vi "Ladder chip&bias ring encapsulation v1.vi"() -> ()   [LabVIEW 2016]
uses:
  Classes/Controllers/Camera/Copy of Controller Folder/Controller.lvclass
  <vilib>/Utility/file.llb/Read Delimited Spreadsheet (DBL).vi
  Classes/Controllers/Motion/Copy of Motion Folder/Motion.lvclass
  Classes/Controllers/Dispenser/Copy of Ultimus V2 Folder/Ultimus V2.lvclass
  Classes/Controllers/I-O/Copy of NI-DAQ Folder/NI-DAQ.lvclass
  <vilib>/Analysis/NI_AALPro.lvlib
  <vilib>/Analysis/coordinate.llb/2D Cartesian Coordinate Rotation (Scalar).vi
  <vilib>/Utility/file.llb/Write Delimited Spreadsheet (DBL).vi
panel:
  out "Needle parking position 2":dbl[](array[numeric])
  out "x+y 2":dbl[](array[numeric])
  out "corner index 2":i32
  in  "Deposit Glue for chip":bool
  out "Measured HDI size":dbl[](array[numeric])
  out "Measured HDI top left mark":dbl[](array[numeric])
  out "Sample on HDI":dbl[][](array[numeric]) format="%#_8g"
  in  "Default HDI size":dbl[](array[numeric])=[24.2991, 231.315, -0.0249987, -3.34415e-05]
  in  "Default HDI alignment \nmark position":dbl[](array[numeric])=[448.231, 973.808, 78.9737, -3.34415e-05]
  in  "Needle gap for real":dbl=1.3
  out "corner index":i32
  out "Array":dbl[](array[numeric])
  out "x+y":dbl[](array[numeric])
  out "CMC positions":dbl[][][](array[numeric])
  in  "deposit module":i32=2
  out "Stave mark":dbl[][](array[numeric])
  in  "Default Stave dimension":dbl[](array[numeric])=[34.0, 472.0, -0.335295, -0.000320234]
  in  "Default Stave upper left mark":dbl[](array[numeric])=[584.376, 675.576, 70.9882, 0.000840064]
  out "Needle parking position":dbl[](array[numeric])
  in  "Uppler / Lower Stave":bool=TRUE
  out "Gantry current position":dbl[](array[numeric])
  in  "READ Position":bool
  in  "Needle Alignment":bool
  in  "Parking position":dbl[](array[numeric])=[625.0, 625.0, 0.0, 0.01]
  in  "GOTO":bool
  out "# of tasks excuted":i32
  in  "Inititalize":bool
  in  "Deposit Glue for bias ring":bool
  in  "Stop":bool
  in  "Measure HDI":bool
  # "Upper\nmodule"
  # "Lower\nmodule"
  # "Chip & Bias ring encapsulation"
  # "Module infomation"
  # "before \"HDI cornrer\" click \"Initialize\""
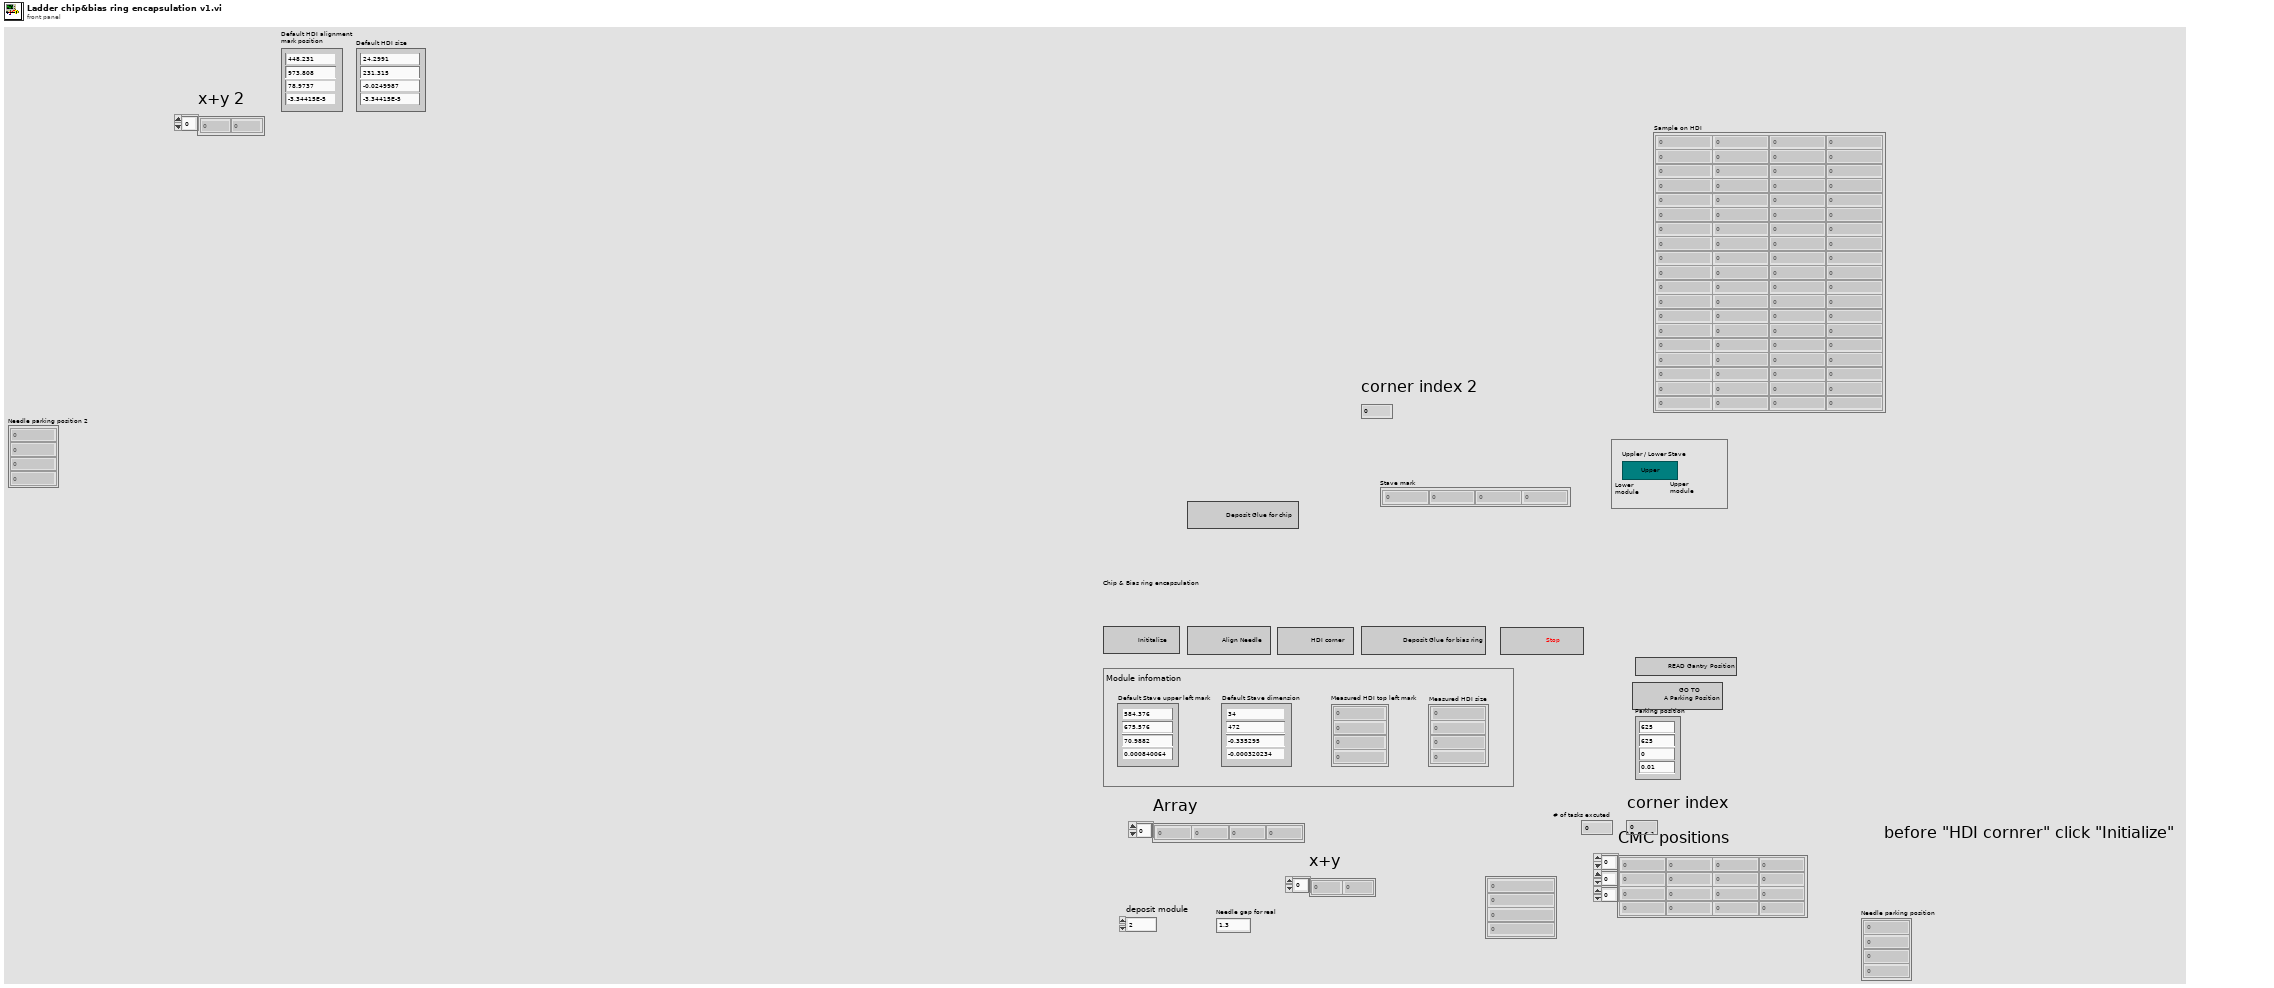
[diagram p1: front panel]
types:
  T1 = typedef "Controller.lvclass/Controllers.ctl" = cluster{"Copy of Motion.lvclass":refnum<class "Motion.lvclass">, "Copy of I-O.lvclass":refnum<class "I-O.lvclass">, "Copy of Dispenser.lvclass":refnum<class "Dispenser.lvclass">}
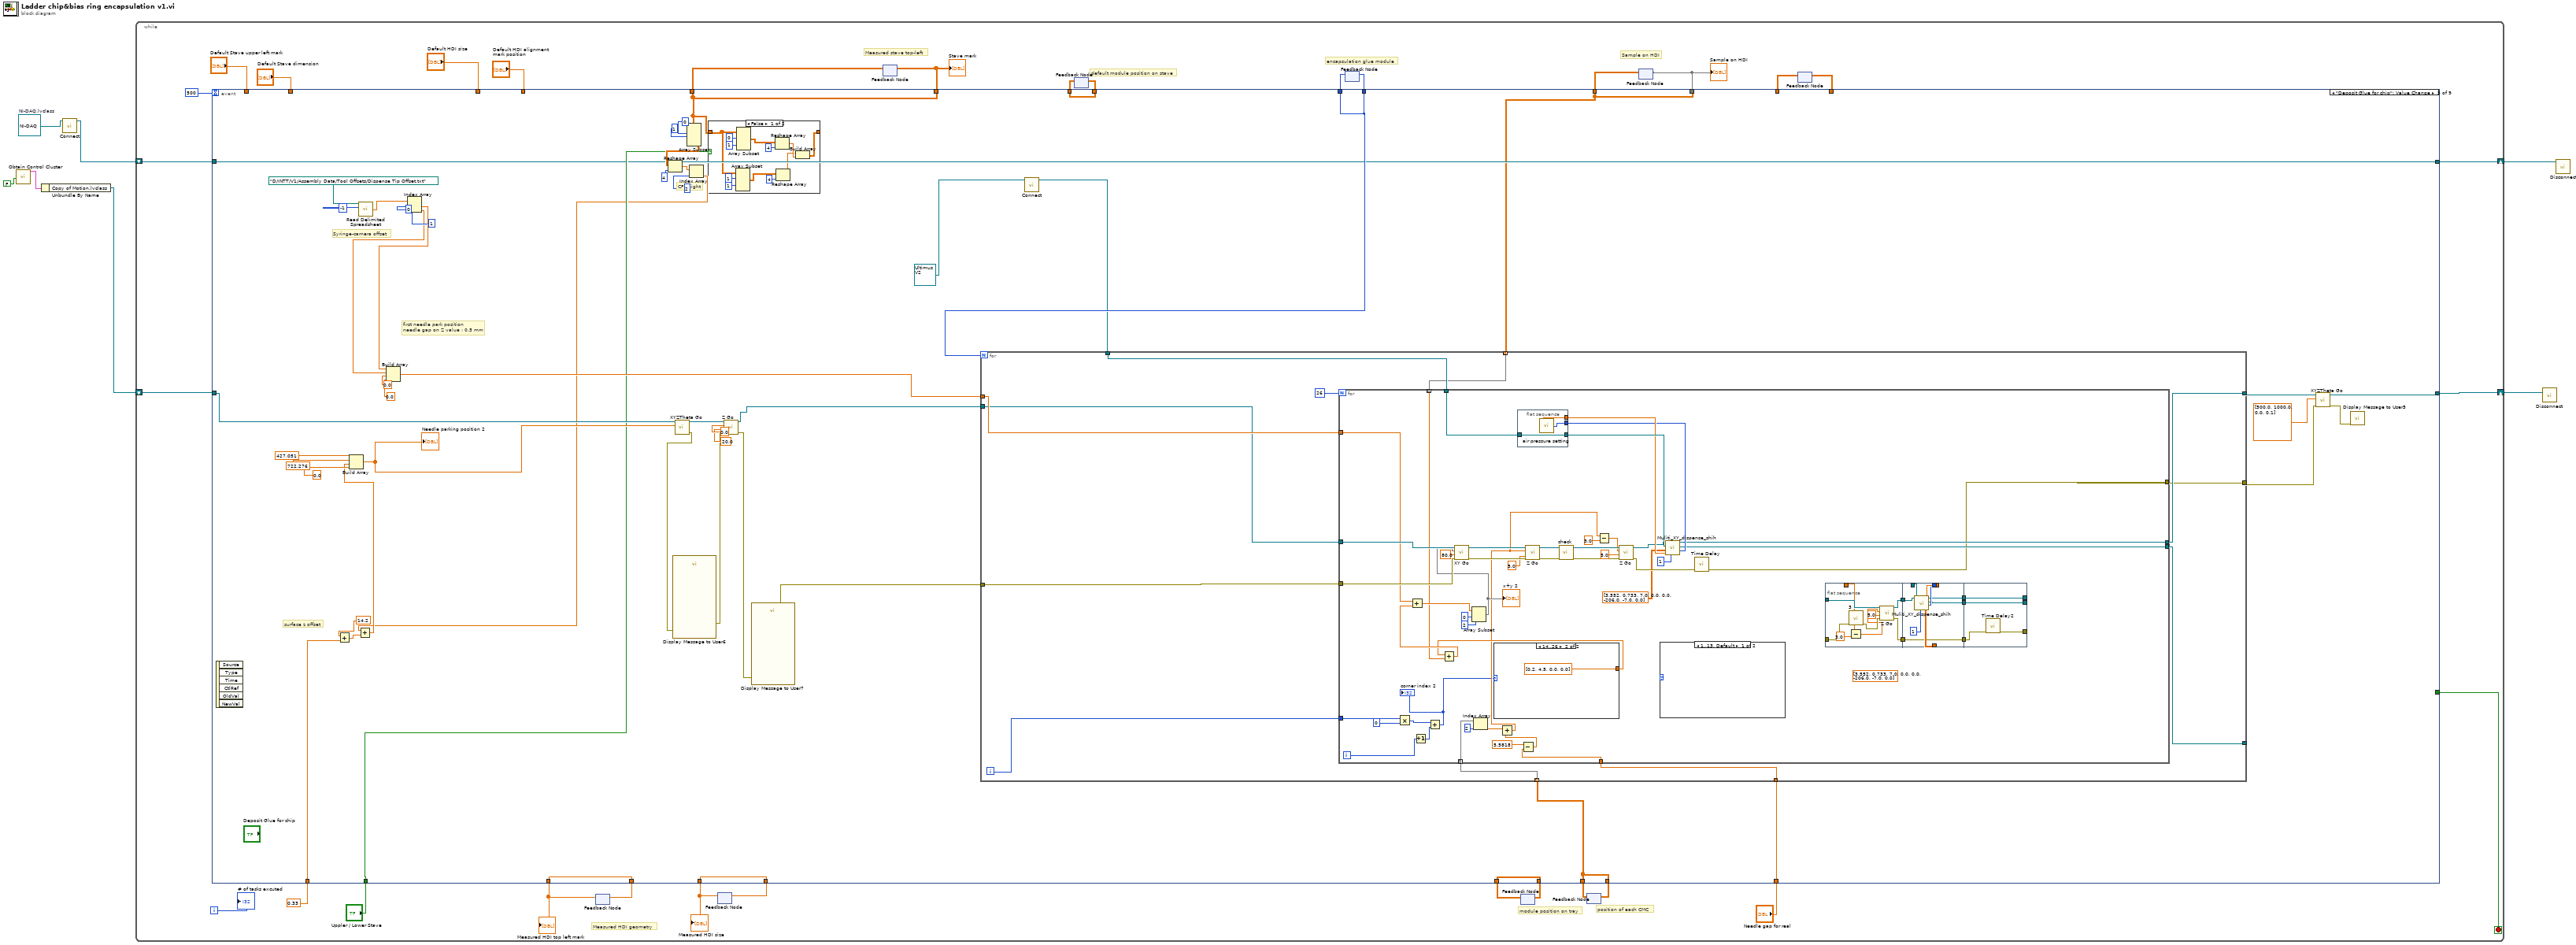
[diagram p0: block diagram]
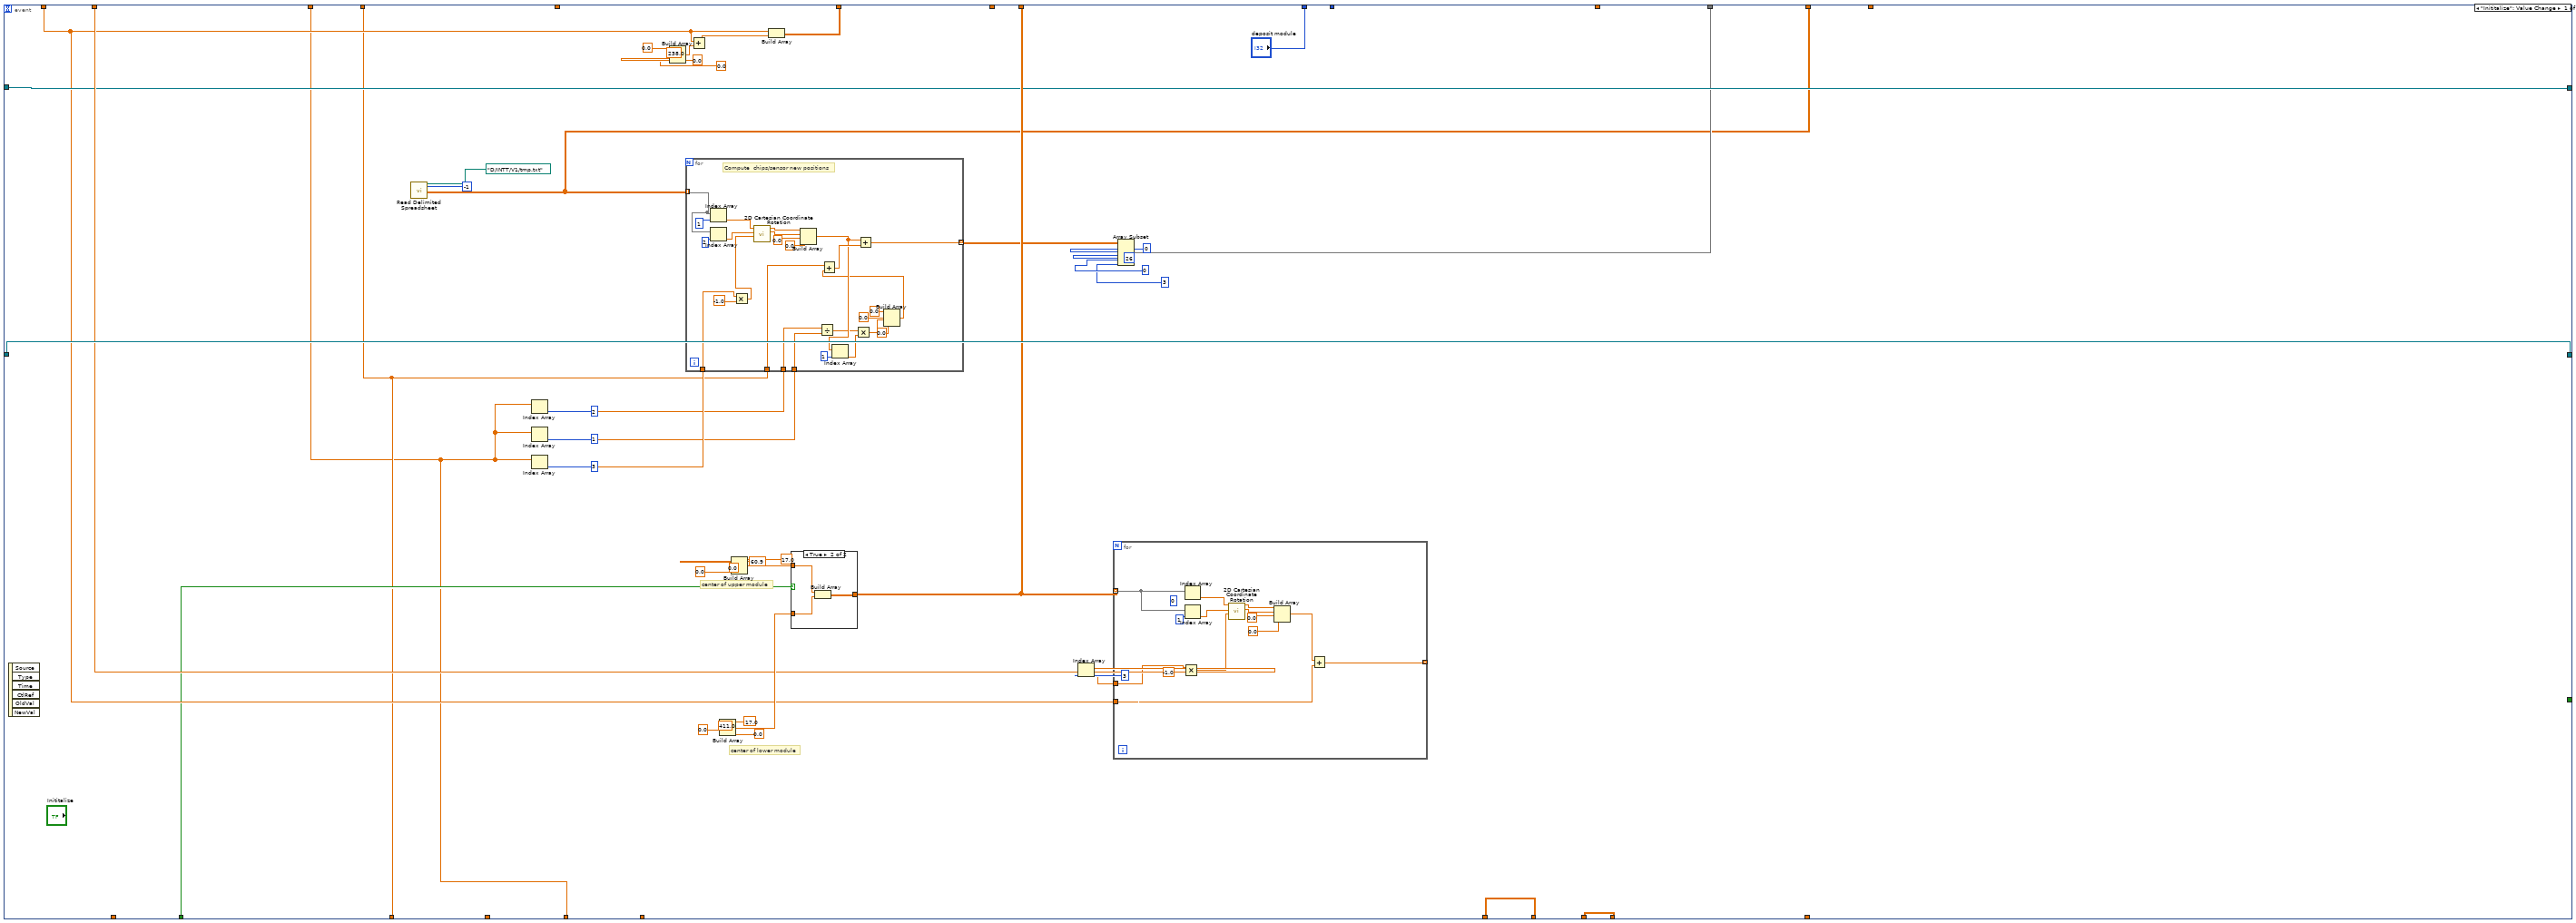
[diagram p2: hidden frame]
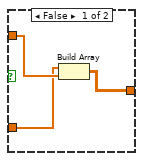
[diagram p3: hidden frame]
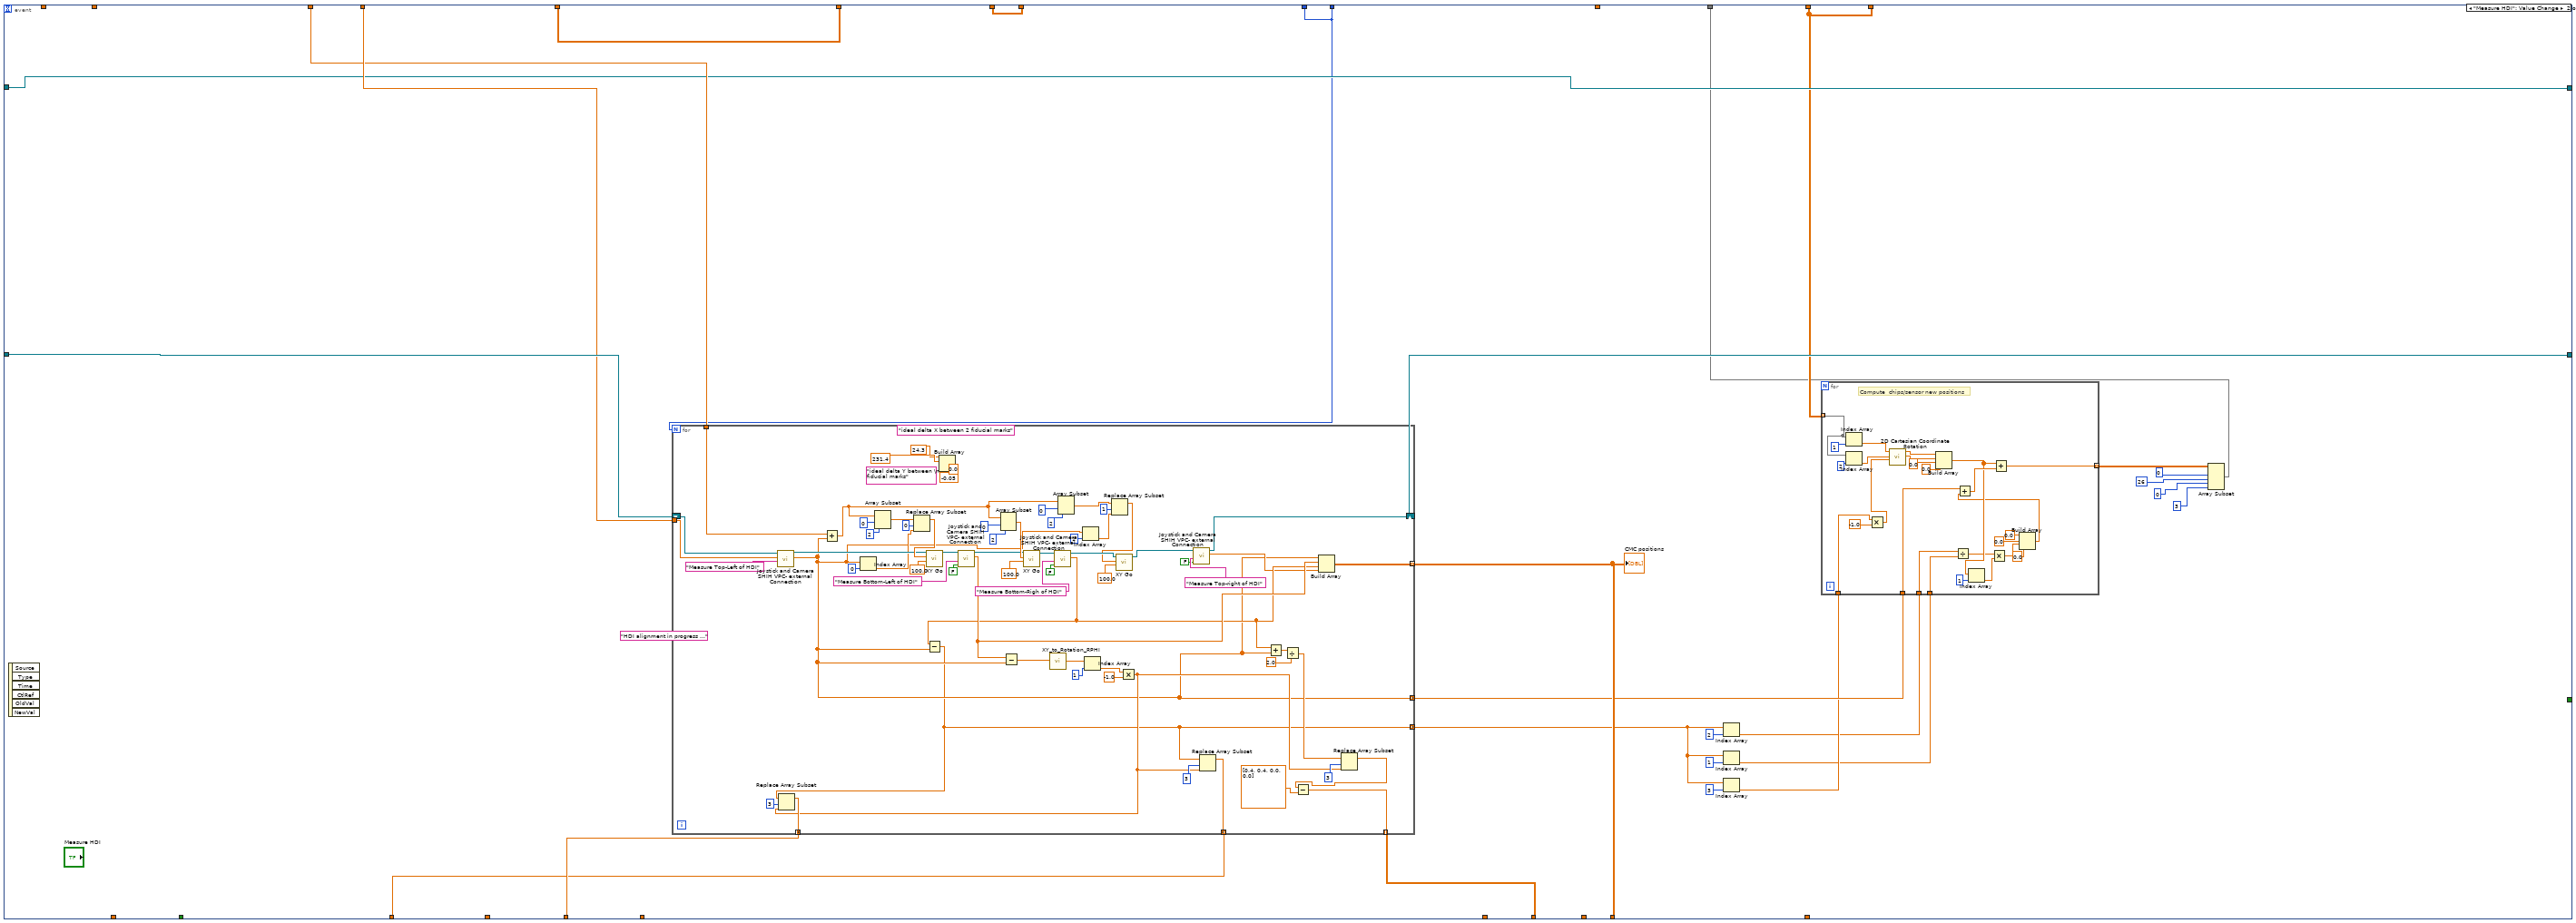
[diagram p4: hidden frame]
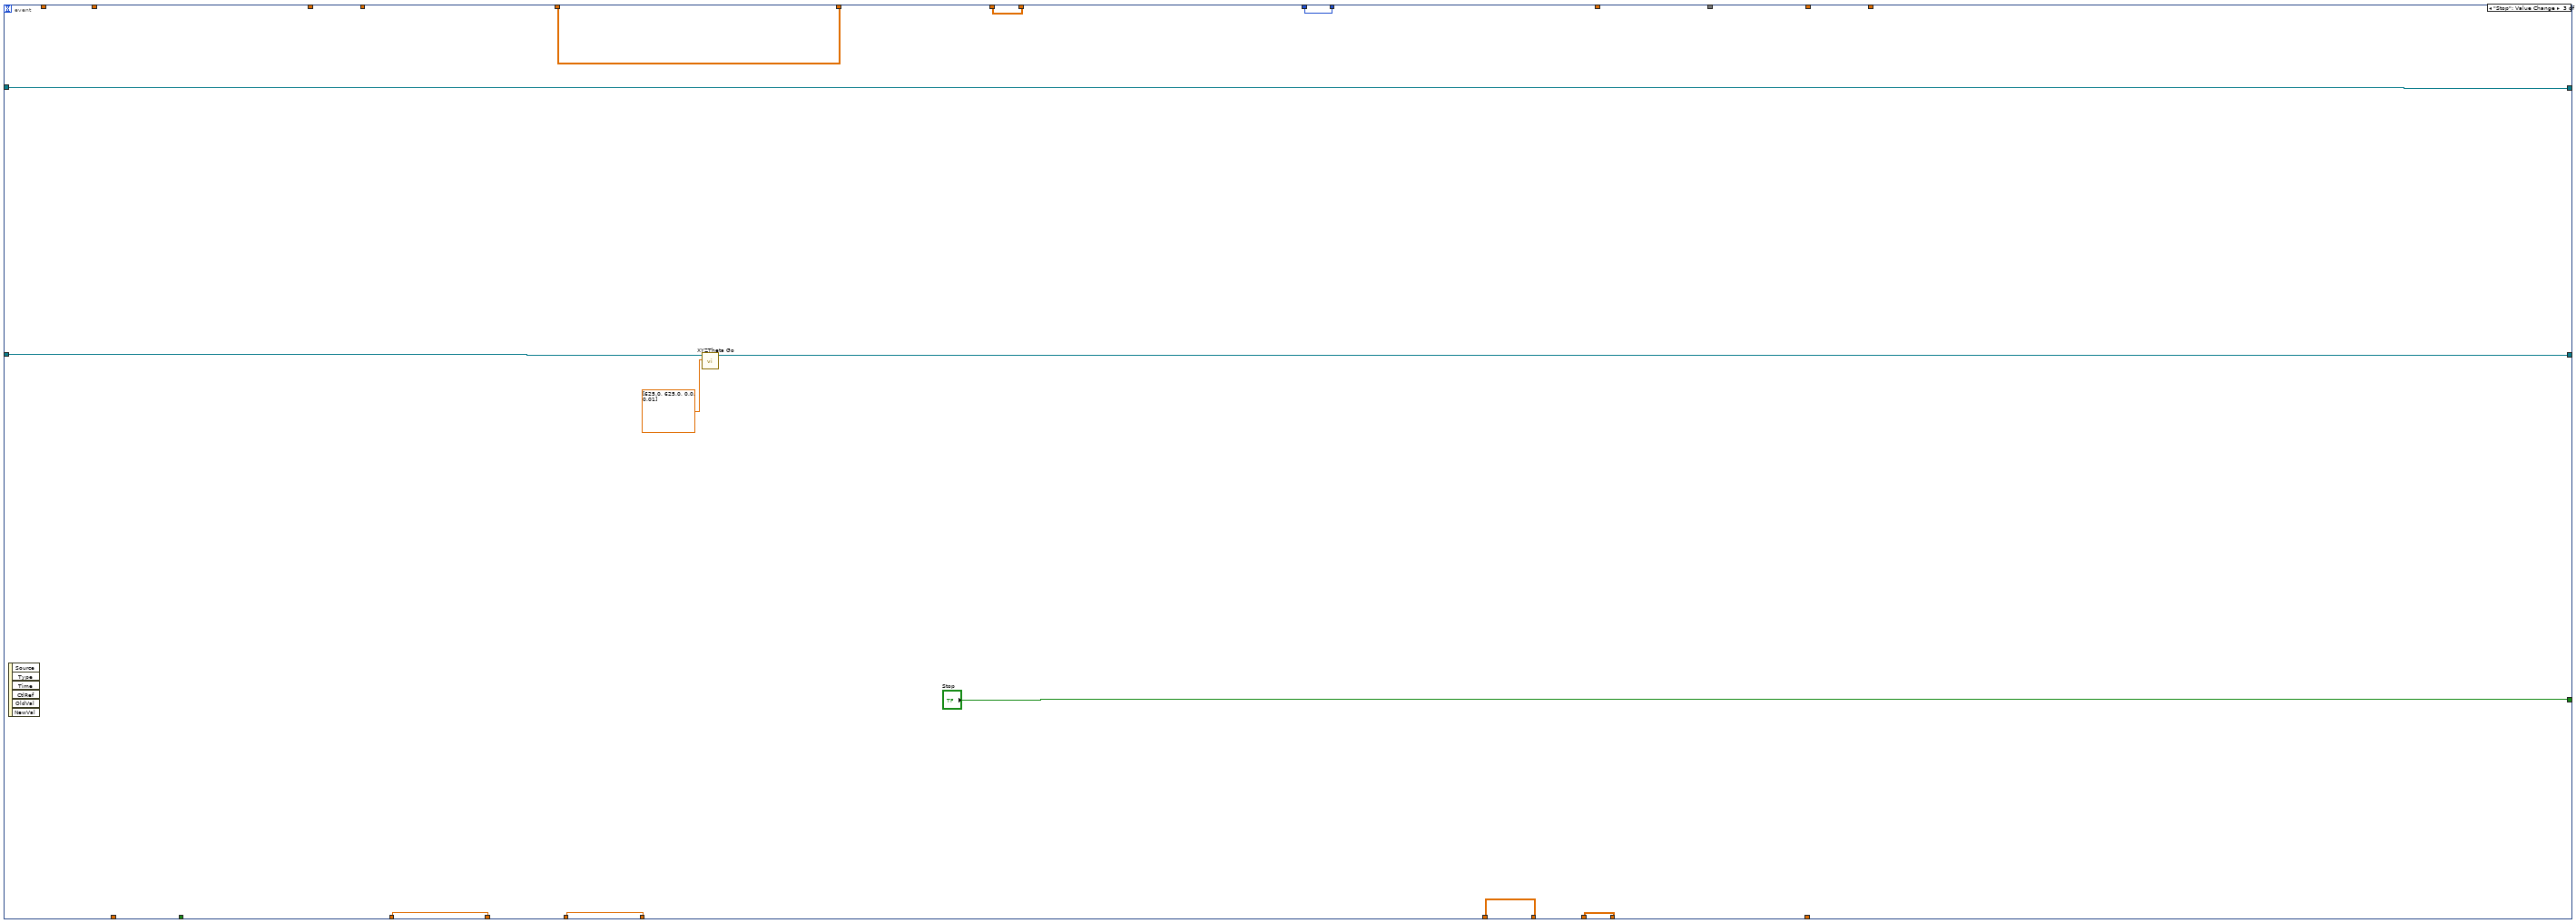
[diagram p5: hidden frame]
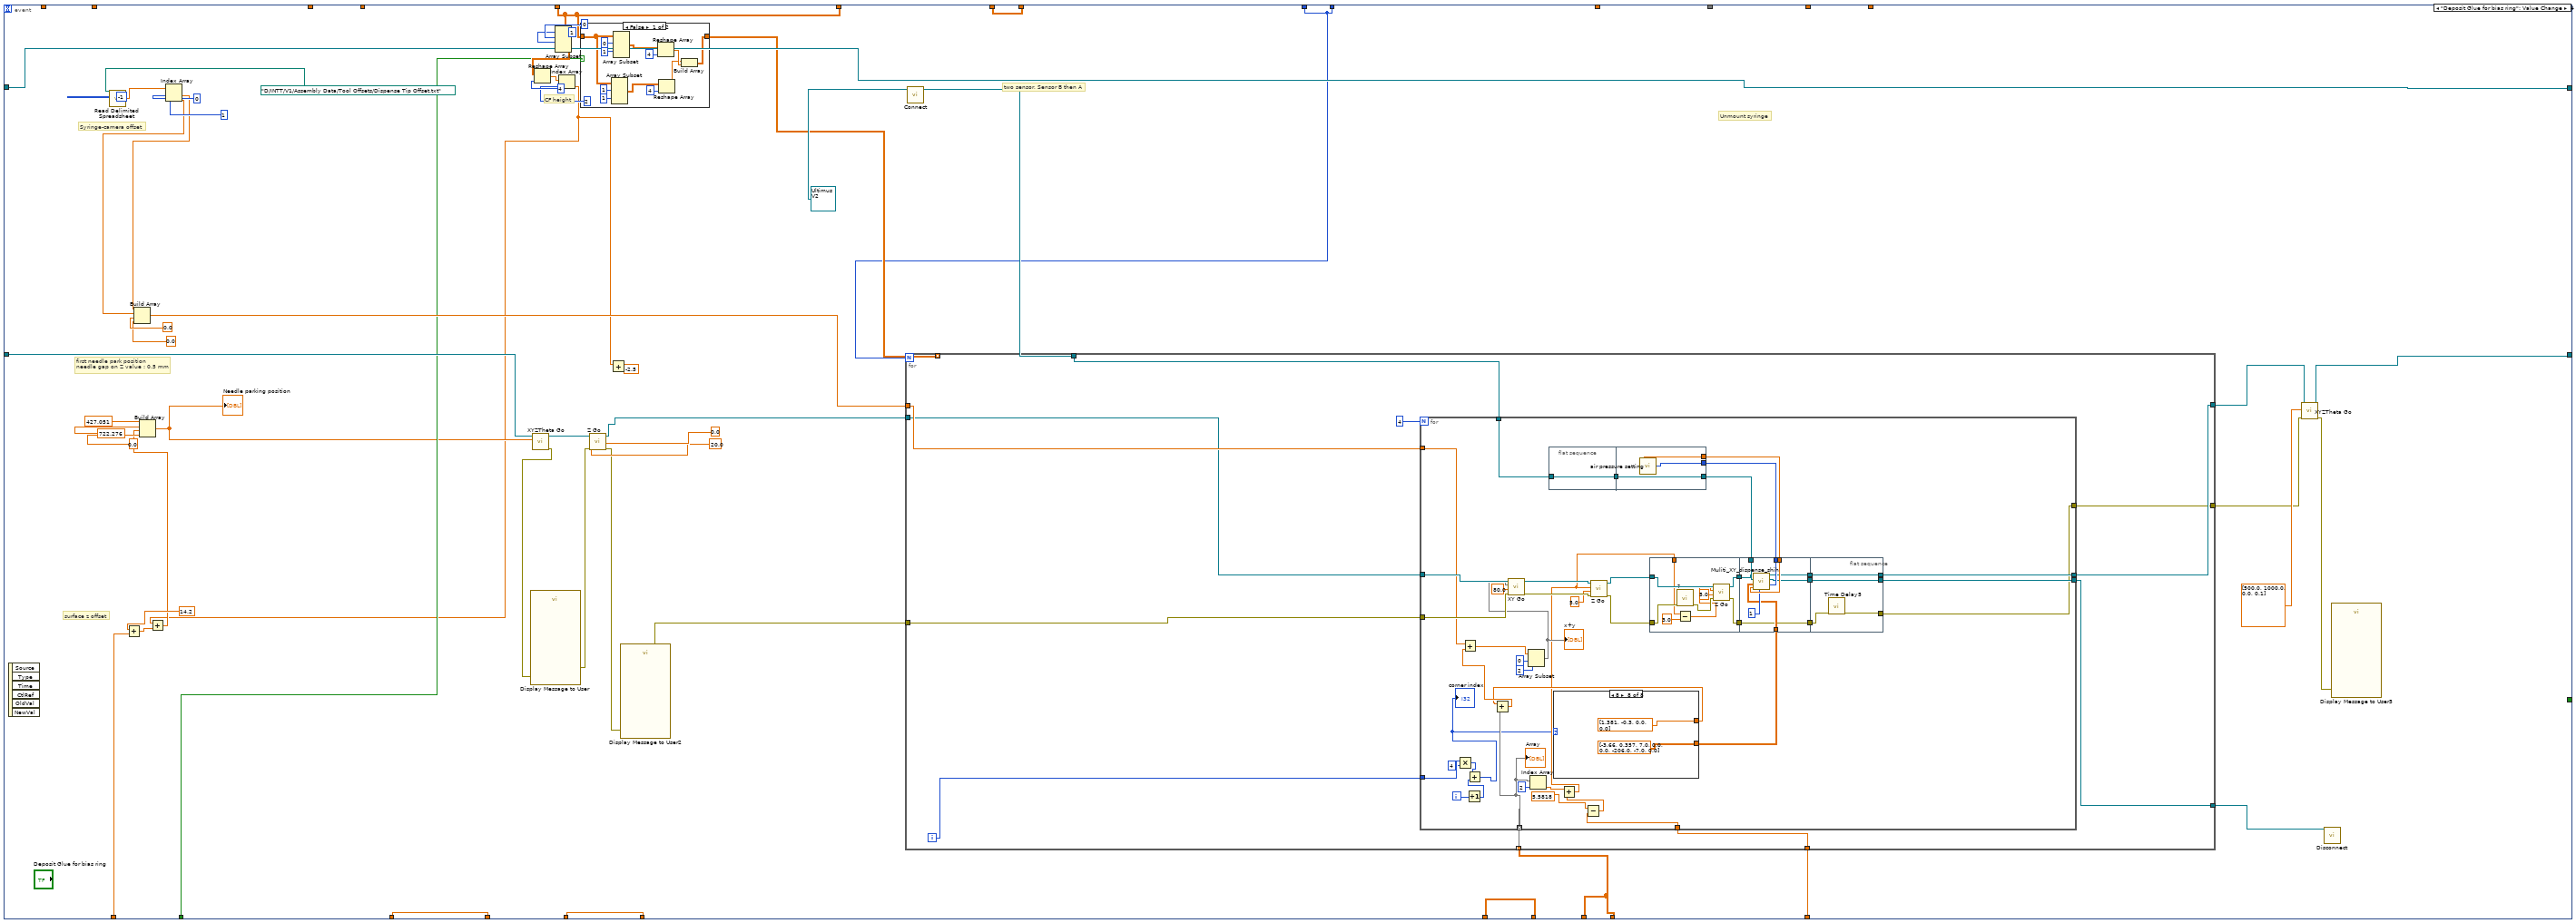
[diagram p6: hidden frame]
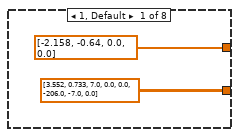
[diagram p8: hidden frame]
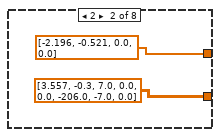
[diagram p9: hidden frame]
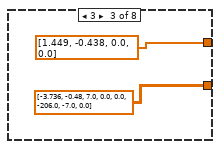
[diagram p10: hidden frame]
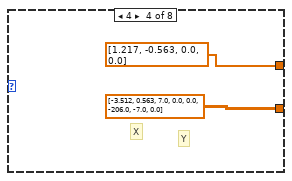
[diagram p11: hidden frame]
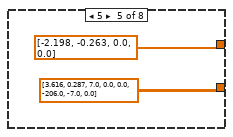
[diagram p12: hidden frame]
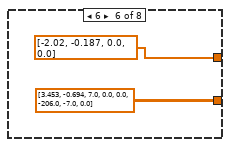
[diagram p13: hidden frame]
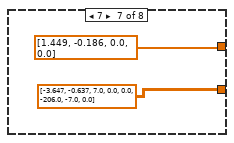
[diagram p14: hidden frame]
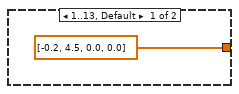
[diagram p17: hidden frame]
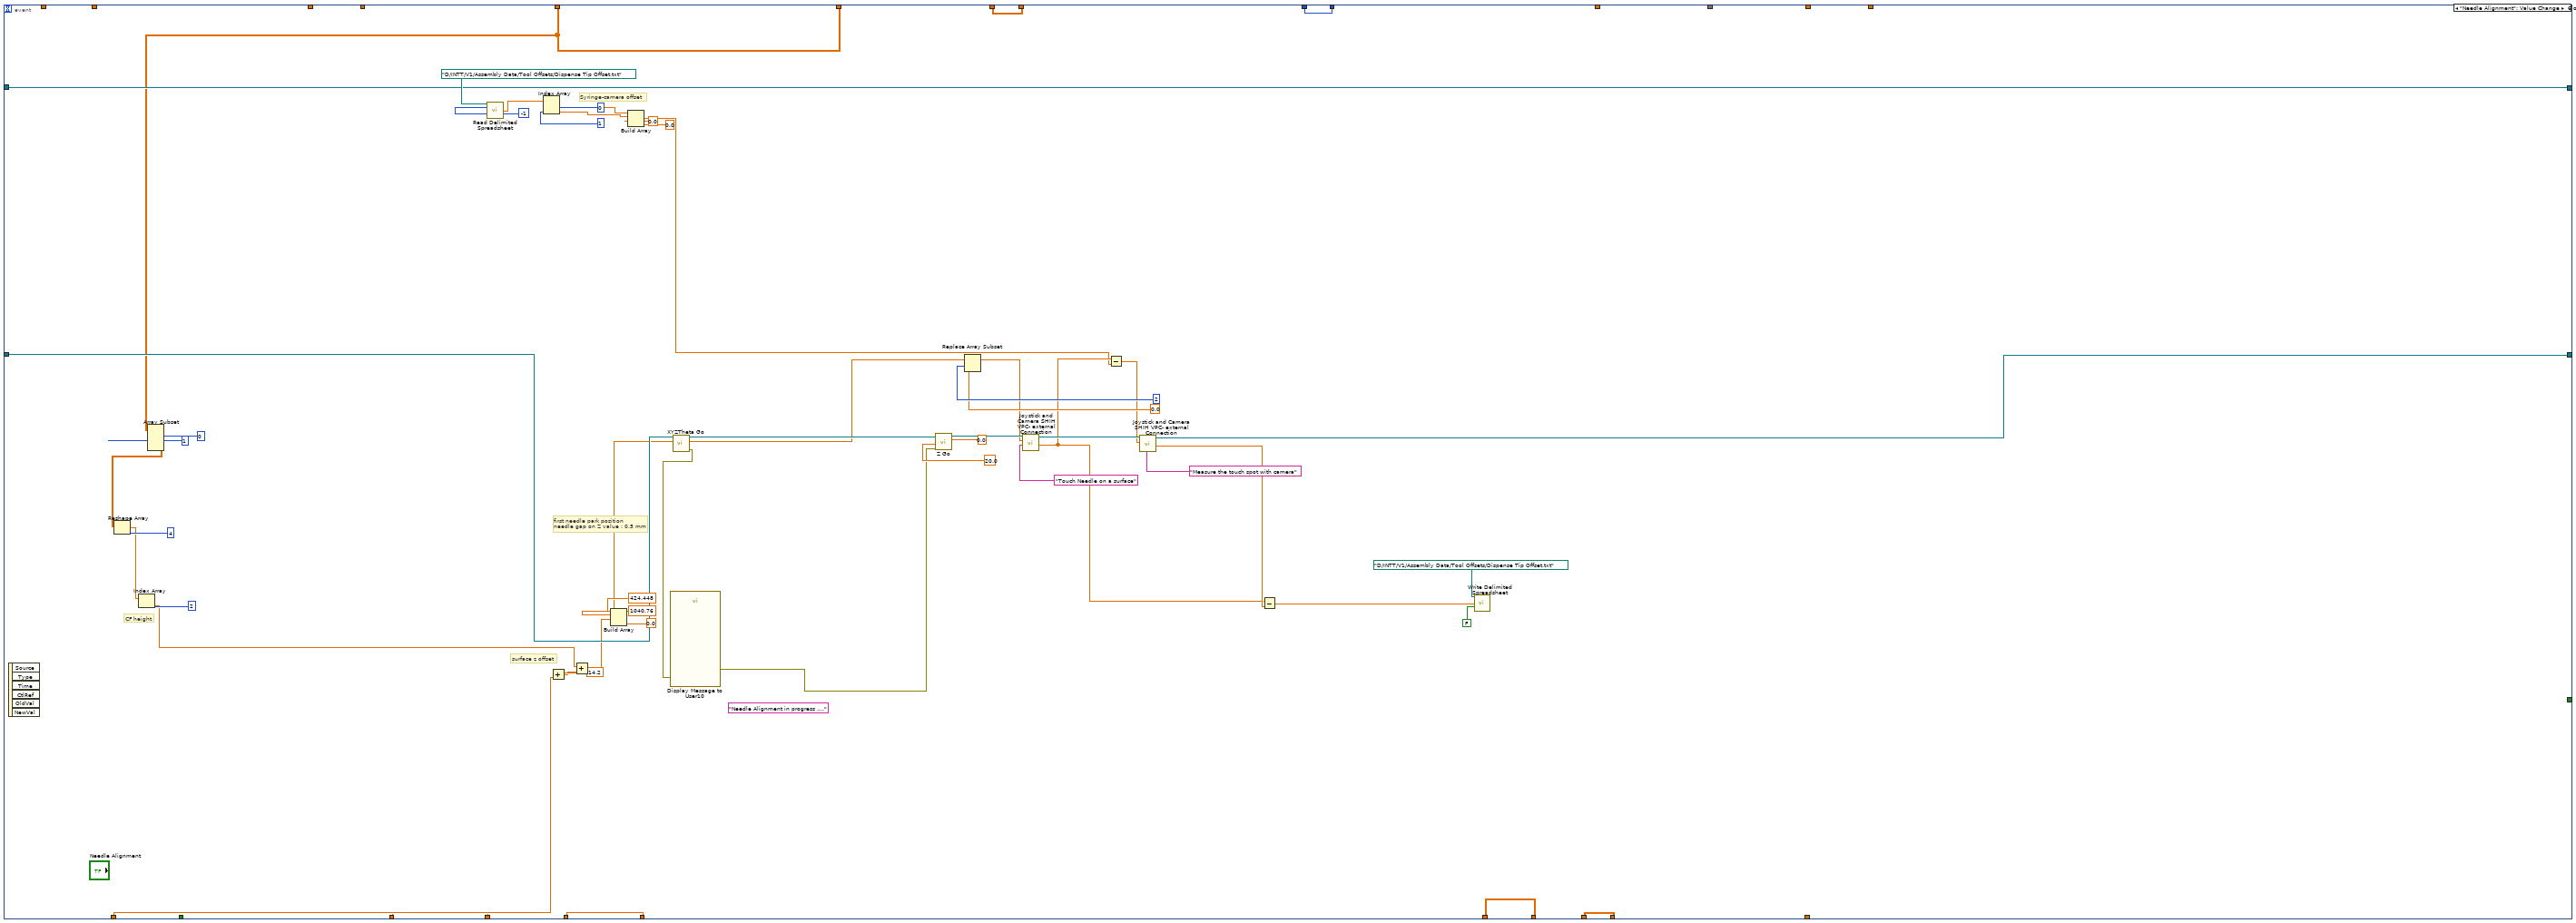
[diagram p18: hidden frame]
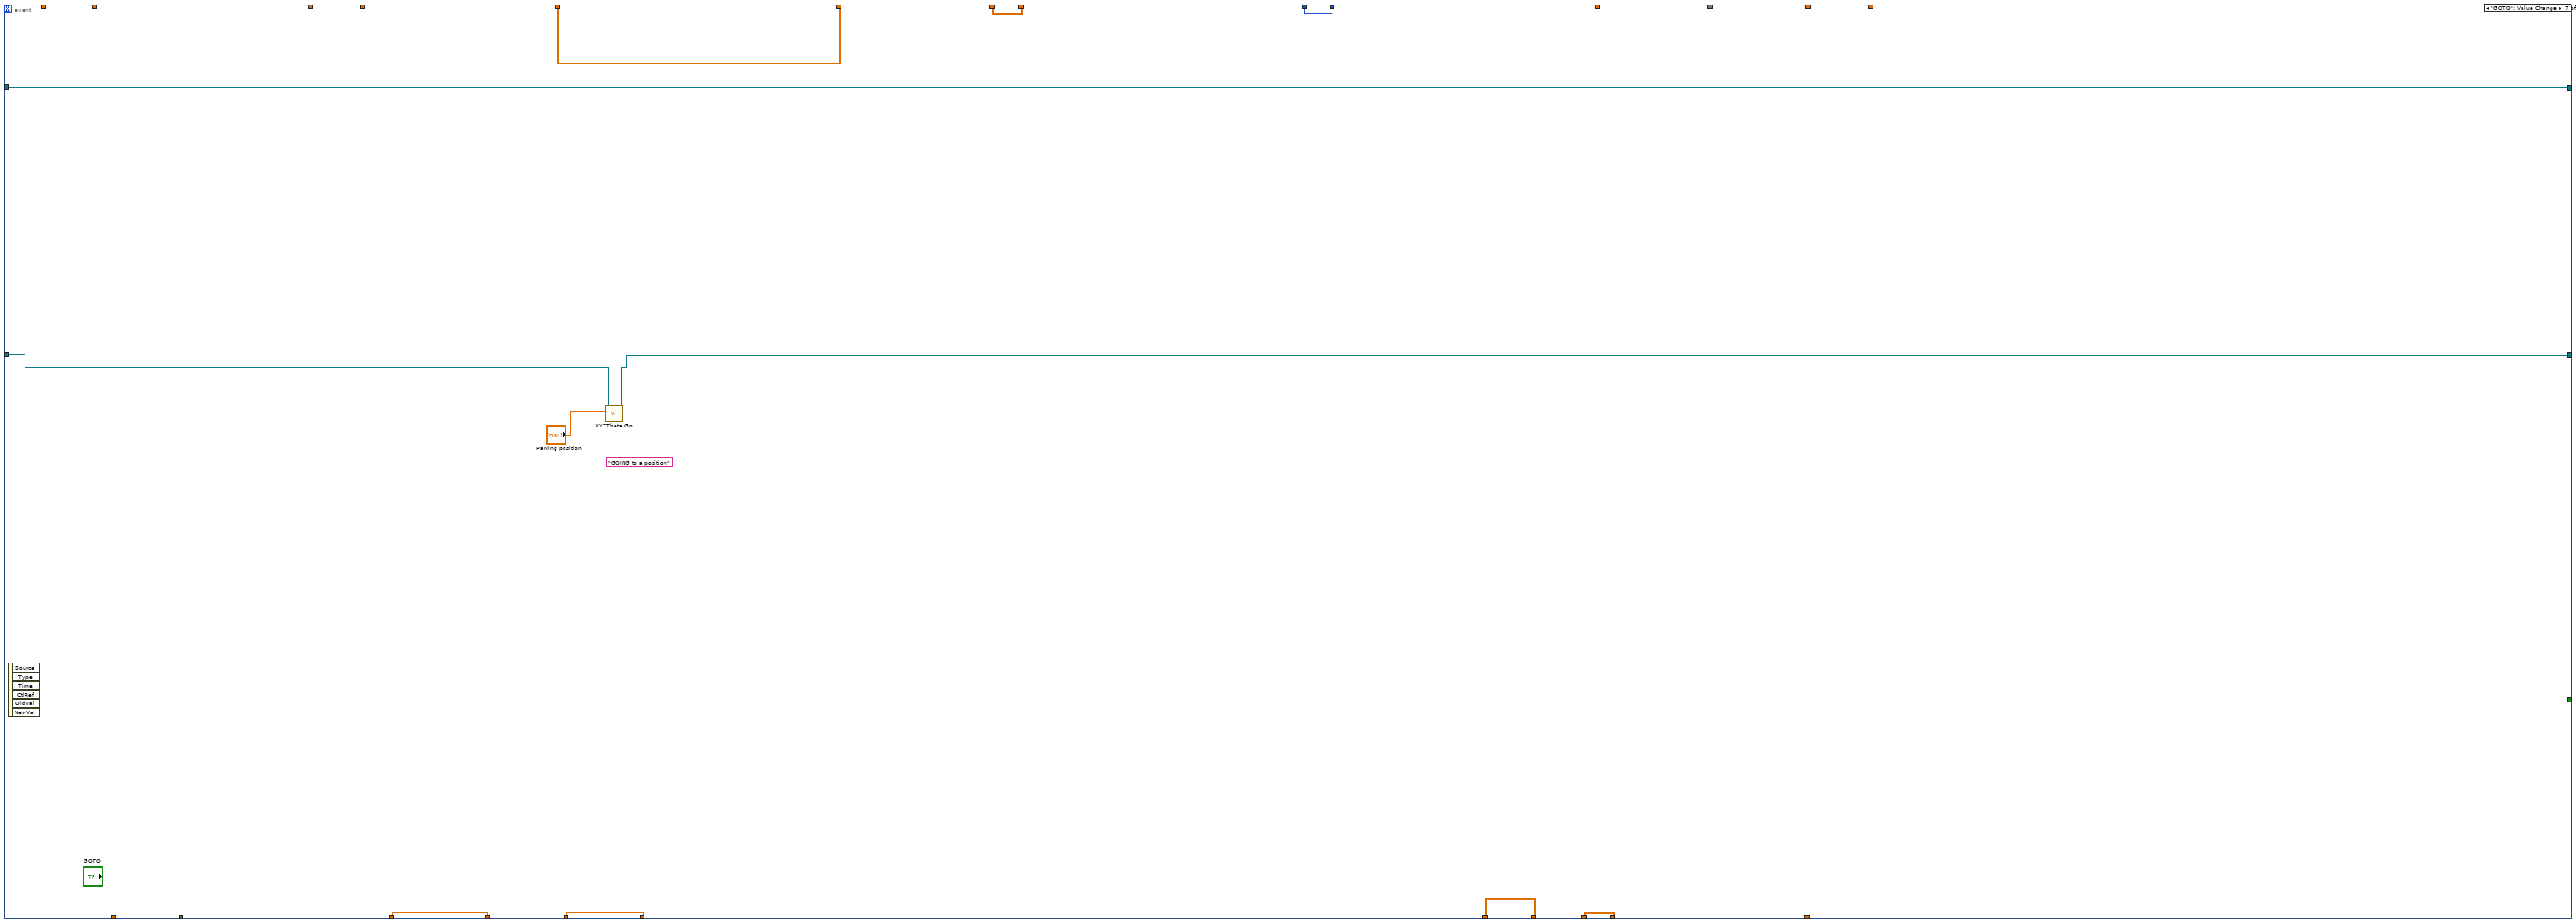
[diagram p19: hidden frame]
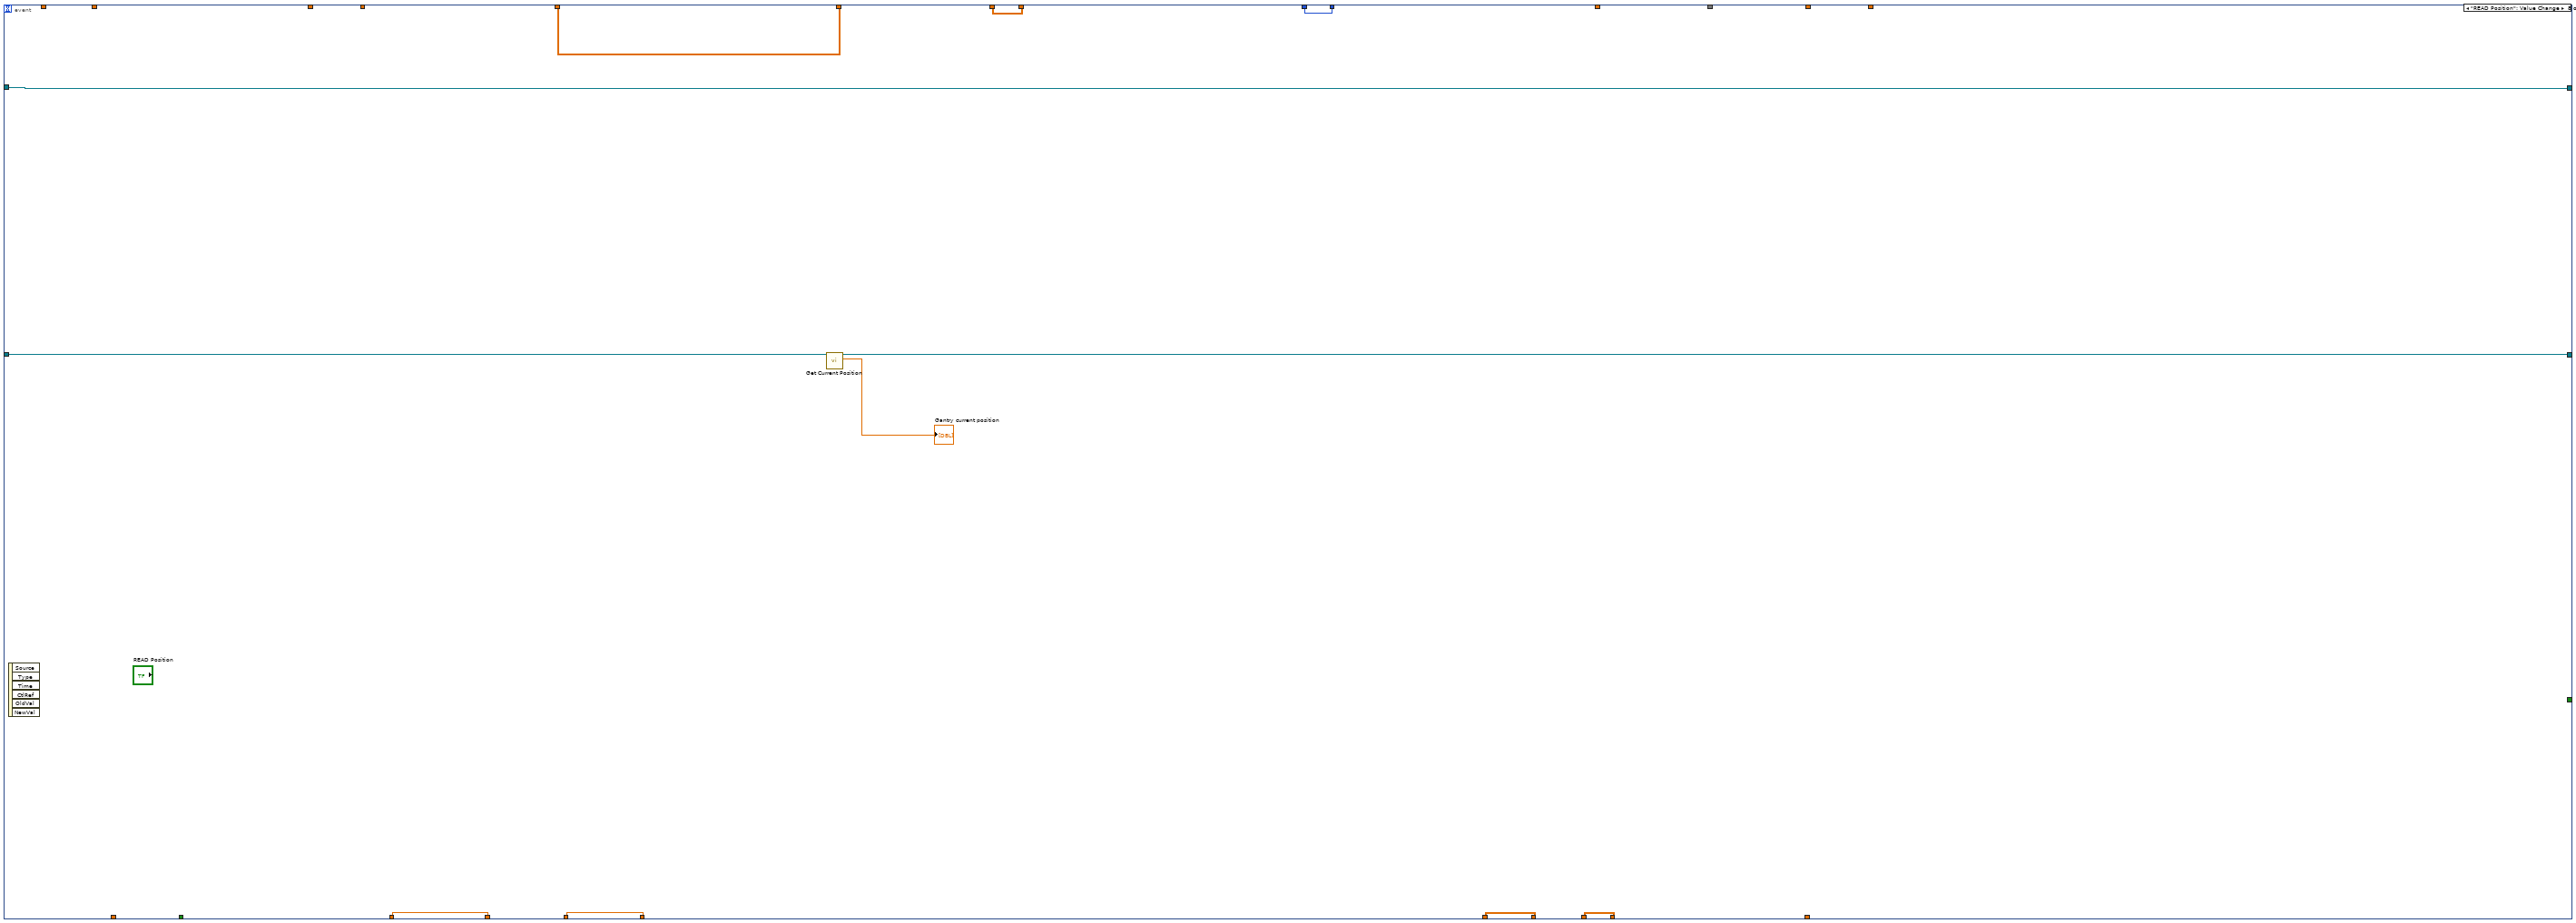
[diagram p20: hidden frame]
diagram:
  w3 = refnum<class "NI-DAQ.lvclass"> refnum  # NI-DAQ.lvclass
  n1 = call "Obtain Control Cluster.vi"("I/O"=FALSE) -> ("Control Out"=w7:T1)  [unwired: 10 in]
  n2 = Unbundle By Name(w7) -> ("Copy of Motion.lvclass"=w5:refnum<class "Motion.lvclass">)
  n3 = call-dynamic "Connect.vi"("NI-DAQ in"=w3) -> ("NI-DAQ out"=w2:refnum<class "NI-DAQ.lvclass">)  [unwired: 9 in, 1 out]
  n4 = while {
    shift-right: [w34] -> w4
    shift-left: w5 -> [w39]
    shift-right: [w24] -> w1
    shift-left: w2 -> [w26]
    i -> [w33]
    stop <- w38 stop-if-true
    # "Sample on HDI"
    # "position of each CMC"
    # "encapsulation glue module"
    # "default module position on stave"
    # "Measured HDI geometry"
    # "module position on tray"
    # "Measured stave top-left"
    n5 = feedback #1() -> (w25:dbl[])  [unwired: 1 in]
    n6 = feedback #2() -> (w36:dbl[])  [unwired: 1 in]
    n7 = feedback #3() -> (w37:dbl[][])  [unwired: 1 in]
    n8 = feedback #4() -> (w31:dbl[][])  [unwired: 1 in]
    n9 = feedback #5() -> (w19:i32)  [unwired: 1 in]
    n10 = feedback #6() -> (w21:dbl[][])  [unwired: 1 in]
    n11 = feedback #7() -> (w17:dbl[][][])  [unwired: 1 in]
    n12 = feedback #8() -> (w12:dbl[][])  [unwired: 1 in]
    n13 = feedback #9() -> (w8:dbl[][])  [unwired: 1 in]
    n14 = event shown="[4] \"Deposit Glue for chip\": Value Change" {
      selector: _ -> [_ _ _ _ _ _ _ _ _]
      dyn-events: _ -> [_ _ _ _ _ _ _ _ _]
      timeout: 500 -> [_ _ _ _ _ _ _ _ _]
      tunnel: w39 -> [w84 w157 w260 w297 w448 w613 w637 w651 w659]
      tunnel: [_ _ "Stop" _ _ _ _ _ _] -> w38
      tunnel: [w60 w152 w256 w269 w434 w581 w640 w648 w658] -> w27
      tunnel: w37 -> [_ w152 w256 w269 w434 w581 w640 w648 w658]
      tunnel: w36 -> [_ _ w249 w261 w425 w576 w630 w641 w653]
      tunnel: [w70 w151 w255 w288 w427 w614 w638 w647 w656] -> w35
      tunnel: w21 -> [w70 _ w255 w288 w427 w614 w638 w647 w656]
      tunnel: [w84 w156 w258 w289 w462 w605 w635 w650 w659] -> w34
      tunnel: "Default HDI alignment \nmark position" -> [w42 w155 _ _ _ _ _ _ _]
      tunnel: "Default HDI size" -> [w41 w154 _ _ _ _ _ _ _]
      tunnel: [w73 w153 w257 w287 w424 w615 w639 w649 w657] -> w32
      tunnel: w31 -> [_ w153 w257 w287 w424 w615 w639 w649 w657]
      tunnel: "Uppler / Lower Stave" -> [w57 _ _ w277 w433 _ _ _ _]
      tunnel: "Default Stave upper left mark" -> [w61 _ _ _ _ _ _ _ _]
      tunnel: "Default Stave dimension" -> [w69 _ _ _ _ _ _ _ _]
      tunnel: w26 -> [w68 w150 w253 w283 w430 w596 w634 w645 w661]
      tunnel: [w68 w150 w253 w283 w430 w596 w634 w645 w660] -> w24
      tunnel: w25 -> [_ _ w250 w262 w426 w577 w631 w642 w652]
      tunnel: 0.33 ("Needle Height Compenstation\n(glue gap)") -> [_ _ _ w278 w431 w589 _ _ _]
      tunnel: ["deposit module" w149 w252 w267 w459 w579 w633 w644 w655] -> w20
      tunnel: w19 -> [_ w149 w252 w267 w459 w579 w633 w644 w655]
      tunnel: [w58 w148 w251 w263 w428 w578 w632 w643 w654] -> w18
      tunnel: w17 -> [w58 _ w251 w263 w428 w578 w632 w643 w654]
      tunnel: "Needle gap for real" -> [_ _ _ w264 w429 _ _ _ _]
      tunnel: [w43 w131 _ _ w423 _ _ _ _] -> w13
      tunnel: w12 -> [_ _ _ _ w423 _ _ _ _]
      tunnel: [w42 w146 w250 w262 w426 w577 w631 w642 w652] -> w11
      tunnel: [w41 w147 w249 w261 w425 w576 w630 w641 w653] -> w10
      tunnel: [w40 w145 _ _ _ _ _ _ _] -> w9
      tunnel: w8 -> [_ w145 _ _ _ _ _ _ _]
      event "Inititalize": Value Change {
        # "center of lower module"
        # "center of upper module"
        n15 = event-data() -> ()  [unwired: 1 in, 6 out]
        n16 = call-poly <vilib>:"Read Delimited Spreadsheet.vi"("file path (dialog if empty)"=path "D:/INTT/V1/tmp.txt", "number of rows (all:-1)"=-1) -> ("all rows"=w40:dbl[][])  [unwired: 8 in, 5 out]
        n17 = Index Array(array=w41, index=2) -> (element=w49:dbl)
        n18 = Index Array(array=w41, index=1) -> (element=w50:dbl)
        n19 = Index Array(array=w41, index=3) -> (element=w51:dbl)
        n20 = Build Array(0.0 ("element"), 238.0 ("element"), 0.0 ("element"), 0.0 ("element")) -> (w63:dbl[])
        n21 = for {
          tunnel: w40 -> [w103] mode=indexing
          tunnel: w51 -> [w88]
          tunnel: w42 -> [w96]
          tunnel: [w102] -> w44 mode=indexing
          tunnel: w49 -> [w101]
          tunnel: w50 -> [w94]
          # "Compute  chips/sensor new positions"
          n22 = Index Array(array=w103, index=1) -> (element=w107:dbl)
          n23 = Index Array(array=w103, index=2) -> (element=w106:dbl)
          n24 = Multiply(x=w88, y=-1.0) -> (x*y=w89:dbl)
          n25 = call-poly <vilib>:"2D Cartesian Coordinate Rotation.vi"("theta"=w89, "y"=w106, "x"=w107) -> ("y out"=w109:dbl, "x out"=w108:dbl)  [unwired: 6 in, 1 out]
          n26 = Build Array(w108, w109, 0.0 ("element"), 0.0 ("element")) -> (w91:dbl[])
          n27 = Divide(x=w101, y=w94) -> (x/y=w85:dbl)
          n28 = Index Array(array=w91, index=1) -> (element=w92:dbl)
          n29 = Multiply(x=w85, y=w92) -> (x*y=w97:dbl)
          n30 = Build Array(0.0 ("element"), 0.0 ("element"), w97, 0.0 ("element")) -> (w86:dbl[])
          n31 = Add(x=w96, y=w86) -> (x+y=w95:dbl[])
          n32 = Add(x=w91, y=w95) -> (x+y=w102:dbl[])
        }
        n33 = Add(x=w61, y=w63) -> (x+y=w62:dbl[])
        n34 = Build Array(17.0 ("element"), 411.0 ("element"), 0.0 ("element"), 0.0 ("element")) -> (w74:dbl[])
        n35 = Build Array(17.0 ("element"), 60.9 ("element"), 0.0 ("element"), 0.0 ("element")) -> (w75:dbl[])
        n36 = Build Array(w61, w62) -> (w60:dbl[][])
        n37 = case shown="True" w57 {
          tunnel: w75 -> [w113 w116]
          tunnel: w74 -> [w112 w115]
          tunnel: [w111 w114] -> w73
          frame False {
            n38 = Build Array(w112, w113) -> (w111:dbl[][])
          }
          frame True {
            n39 = Build Array(w116, w115) -> (w114:dbl[][])
          }
        }
        n40 = Index Array(array=w69, index=3) -> (element=w71:dbl)
        n41 = for {
          tunnel: w73 -> [w124] mode=indexing
          tunnel: w71 -> [w118]
          tunnel: w61 -> [w123]
          tunnel: [w121] -> _ mode=indexing
          (unwired) 0 ("index")
          n42 = Multiply(x=w118, y=-1.0) -> (x*y=w119:dbl)
          n43 = Index Array(array=w124) -> (element=w127:dbl)  [unwired: 1 in]
          n44 = Index Array(array=w124, index=1) -> (element=w126:dbl)
          n45 = call-poly <vilib>:"2D Cartesian Coordinate Rotation.vi"("theta"=w119, "y"=w126, "x"=w127) -> ("y out"=w129:dbl, "x out"=w128:dbl)  [unwired: 6 in, 1 out]
          n46 = Build Array(w128, w129, 0.0 ("element"), 0.0 ("element")) -> (w122:dbl[])
          n47 = Add(x=w122, y=w123) -> (x+y=w121:dbl[])
        }
        n48 = Array Subset(array=w44, index (row)=0 ("index"), length (row)=26 ("length"), index (col)=0, length (col)=3 ("length")) -> (w43:dbl[][])
      }
      event "Measure HDI": Value Change {
        (unwired) "HDI alignment in progress ..." ("String")
        n49 = event-data() -> ()  [unwired: 1 in, 6 out]
        n50 = for {
          N: w149 -> [_]
          tunnel: w154 -> [w213]
          shift-right: [w203] -> w156
          shift-left: w157 -> [w211]
          tunnel: w155 -> [w212]
          tunnel: [w245] -> w146 mode=concatenating
          tunnel: [w244] -> w147 mode=concatenating
          tunnel: [w204] -> w151 mode=indexing
          tunnel: [w186] -> w148 mode=indexing
          tunnel: [w185] -> w144 mode=concatenating
          tunnel: [w184] -> w140 mode=concatenating
          (unwired) "ideal delta Y between \n2 fiducial marks"
          (unwired) "ideal delta X between 2 fiducial marks"
          n51 = call "Joystick and Camera SHIH VPC- external Connection.vi"("Motion in"=w211, "XYZTheta"=w212, "Measurement Point"="Measure Top-Left of HDI") -> ("Motion out"=w225:refnum<class "Motion.lvclass">, "Sum"=w185:dbl[])  [unwired: 4 in, 2 out]
          n52 = Add(x=w213, y=w185) -> (x+y=w196:dbl[])
          n53 = Index Array(array=w185, index=0) -> (element=w216:dbl)
          n54 = Array Subset(array=w196, index=0, length=2) -> (w228:dbl[])
          n55 = Replace Array Subset(array=w228, new element=w216, index=0) -> (w226:dbl[])
          n56 = call-dynamic "XY Go.vi"("Speed"=100.0, "XY"=w226, "Motion in"=w225) -> ("Motion out"=w232:refnum<class "Motion.lvclass">)  [unwired: 7 in, 1 out]
          n57 = Build Array(24.3 ("y"), 231.4 ("y"), 0.0 ("element"), -0.05 ("element")) -> ()  [unwired: 1 out]
          n58 = call "Joystick and Camera SHIH VPC- external Connection.vi"("Motion in"=w232, "Measurement Point"="Measure Bottom-Left of HDI", "Inital GO"=FALSE) -> ("Motion out"=w224:refnum<class "Motion.lvclass">, "Sum"=w189:dbl[])  [unwired: 4 in, 2 out]
          n59 = Array Subset(array=w196, index=0, length=2) -> (w238:dbl[])
          n60 = Subtract(x=w189, y=w185) -> (x-y=w223:dbl[])
          n61 = call-dynamic "XY Go.vi"("Speed"=100.0, "XY"=w238, "Motion in"=w224) -> ("Motion out"=w242:refnum<class "Motion.lvclass">)  [unwired: 7 in, 1 out]
          n62 = call "XY_to_Rotation_RPHI.vi"("X-Y"=w223) -> ("r-phi"=w219:dbl[])
          n63 = call "Joystick and Camera SHIH VPC- external Connection.vi"("Motion in"=w242, "Measurement Point"="Measure Bottom-Righ of HDI", "Inital GO"=FALSE) -> ("Motion out"=w201:refnum<class "Motion.lvclass">, "Sum"=w188:dbl[])  [unwired: 4 in, 2 out]
          n64 = Subtract(x=w188, y=w185) -> (x-y=w184:dbl[])
          n65 = Array Subset(array=w196, index=0, length=2) -> (w192:dbl[])
          n66 = Index Array(array=w185, index=1) -> (element=w193:dbl)
          n67 = Index Array(array=w219, index=1) -> (element=w214:dbl)
          n68 = Replace Array Subset(array=w192, new element=w193, index=1) -> (w191:dbl[])
          n69 = call-dynamic "XY Go.vi"("Speed"=100.0, "XY"=w191, "Motion in"=w201) -> ("Motion out"=w200:refnum<class "Motion.lvclass">)  [unwired: 7 in, 1 out]
          n70 = Multiply(x=w214, y=-1.0) -> (x*y=w208:dbl)
          n71 = Replace Array Subset(array=w184, new element=w208, index=3) -> (w244:dbl[])
          n72 = call "Joystick and Camera SHIH VPC- external Connection.vi"("Motion in"=w200, "Measurement Point"="Measure Top-right of HDI", "Inital GO"=FALSE) -> ("Motion out"=w203:refnum<class "Motion.lvclass">, "Sum"=w187:dbl[])  [unwired: 4 in, 2 out]
          n73 = Replace Array Subset(array=w184, new element=w208, index=3) -> (w245:dbl[])
          n74 = Add(x=w188, y=w185) -> (x+y=w247:dbl[])
          n75 = Divide(x=w247, y=2.0) -> (x/y=w207:dbl[])
          n76 = Build Array(w185, w189, w188, w187) -> (w186:dbl[][])
          n77 = Replace Array Subset(array=w207, new element=w208, index=3) -> (w205:dbl[])
          n78 = Subtract(x=w205, y=dbl[] [0.4, 0.4, 0.0, 0.0]) -> (x-y=w204:dbl[])
        }
        "CMC positions" <- w148
        n79 = Index Array(array=w140, index=2) -> (element=w137:dbl)
        n80 = Index Array(array=w140, index=1) -> (element=w138:dbl)
        n81 = Index Array(array=w140, index=3) -> (element=w139:dbl)
        n82 = for {
          tunnel: w145 -> [w176] mode=indexing
          tunnel: w139 -> [w161]
          tunnel: w144 -> [w169]
          tunnel: [w175] -> w132 mode=indexing
          tunnel: w137 -> [w174]
          tunnel: w138 -> [w167]
          # "Compute  chips/sensor new positions"
          n83 = Index Array(array=w176, index=1) -> (element=w180:dbl)
          n84 = Index Array(array=w176, index=2) -> (element=w179:dbl)
          n85 = Multiply(x=w161, y=-1.0) -> (x*y=w162:dbl)
          n86 = call-poly <vilib>:"2D Cartesian Coordinate Rotation.vi"("theta"=w162, "y"=w179, "x"=w180) -> ("y out"=w182:dbl, "x out"=w181:dbl)  [unwired: 6 in, 1 out]
          n87 = Build Array(w181, w182, 0.0 ("element"), 0.0 ("element")) -> (w164:dbl[])
          n88 = Divide(x=w174, y=w167) -> (x/y=w158:dbl)
          n89 = Index Array(array=w164, index=1) -> (element=w165:dbl)
          n90 = Multiply(x=w158, y=w165) -> (x*y=w170:dbl)
          n91 = Build Array(0.0 ("element"), 0.0 ("element"), w170, 0.0 ("element")) -> (w159:dbl[])
          n92 = Add(x=w169, y=w159) -> (x+y=w168:dbl[])
          n93 = Add(x=w164, y=w168) -> (x+y=w175:dbl[])
        }
        n94 = Array Subset(array=w132, index (row)=0 ("index"), length (row)=26 ("length"), index (col)=0, length (col)=3 ("length")) -> (w131:dbl[][])
      }
      event "Stop": Value Change {
        n95 = event-data() -> ()  [unwired: 1 in, 6 out]
        n96 = call "XYZTheta Go.vi"("XYZTheta In"=dbl[] [625.0, 625.0, 0.0, 0.01], "Motion in"=w260) -> ("Motion out"=w258:refnum<class "Motion.lvclass">)  [unwired: 7 in, 2 out]
      }
      event "Deposit Glue for bias ring": Value Change {
        # "CF height"
        # "surface z offset"
        # "two sensor, Sensor B then A"
        # "Unmount syringe"
        # "first needle park position\nneedle gap on Z value : 0.5 mm"
        # "Syringe-camera offset"
        n97 = event-data() -> ()  [unwired: 1 in, 6 out]
        n98 = call-poly <vilib>:"Read Delimited Spreadsheet.vi"("file path (dialog if empty)"=path "D:/INTT/V1/Assembly Data/Tool Offsets/Dispense Tip Offset.txt", "number of rows (all:-1)"=-1) -> ("first row"=w310:dbl[])  [unwired: 8 in, 5 out]
        n99 = Add(x=14.2 ("element"), y=w278) -> (x+y=w273:dbl)
        n100 = Index Array(array=w310, index #1=0 ("index"), index #2=1 ("index")) -> (element #1=w305:dbl, element #2=w303:dbl)
        n101 = Build Array(w305, w303, 0.0 ("element"), 0.0 ("element")) -> (w294:dbl[])
        n102 = Array Subset(array=w269, index (row)=0, length (row)=1 ("length")) -> (w279:dbl[][])  [unwired: 2 in]
        n103 = Reshape Array(w279, 4 ("dimension size")) -> (w275:dbl[])
        n104 = Index Array(array=w275, index=2) -> (element=w270:dbl)
        n105 = Add(x=w270, y=w273) -> (x+y=w272:dbl)
        n106 = Build Array(427.051, 722.276, w272, 0.0 ("element")) -> (w271:dbl[])
        "Needle parking position" <- w271
        n107 = call "XYZTheta Go.vi"("XYZTheta In"=w271, "Motion in"=w297) -> ("error out"=w302:errorcluster, "Motion out"=w296:refnum<class "Motion.lvclass">)  [unwired: 7 in, 1 out]
        n108 = call "Display Message to User"("error in (no error)"=w302) -> ("error out"=w298:errorcluster)  [unwired: 9 in, 1 out]
        n109 = case shown="False" w277 {
          tunnel: w269 -> [w318 w327]
          tunnel: [w315 w327] -> w276
          frame False {
            n110 = Array Subset(array=w318, index (row)=1 ("index"), length (row)=1 ("length")) -> (w319:dbl[][])  [unwired: 2 in]
            n111 = Array Subset(array=w318, index (row)=0 ("index"), length (row)=1 ("length")) -> (w322:dbl[][])  [unwired: 2 in]
            n112 = Reshape Array(w322, 4 ("dimension size")) -> (w317:dbl[])
            n113 = Reshape Array(w319, 4 ("dimension size")) -> (w316:dbl[])
            n114 = Build Array(w316, w317) -> (w315:dbl[][])
          }
          frame True {
          }
        }
        n115 = call-dynamic "Z Go.vi"("error in (no error)"=w298, "Speed"=20.0, "Position"=0.0, "Motion in"=w296) -> ("error out"=w295:errorcluster, "Motion out"=w266:refnum<class "Motion.lvclass">)  [unwired: 6 in]
        n116 = Add(x=w270, y=-2.5) -> ()  [unwired: 1 out]
        n117 = call "Display Message to User2"("error in (no error)"=w295) -> ("error out"=w265:errorcluster)  [unwired: 9 in, 1 out]
        n118 = call-dynamic "Connect.vi"("Ultimus V in"=refnum<class "Ultimus V2.lvclass"> refnum ("Ultimus V2.lvclass")) -> ("Ultimus V out"=w293:refnum<class "Ultimus V2.lvclass">)  [unwired: 9 in, 1 out]
        n119 = for {
          N: w267 -> [_]
          tunnel: w293 -> [w337]
          tunnel: w294 -> [w332]
          tunnel: w276 -> [_] mode=indexing
          tunnel: [w335] -> w285
          tunnel: [w334] -> w284
          tunnel: w265 -> [w330]
          tunnel: [w333] -> w268
          tunnel: w263 -> [w336] mode=indexing
          tunnel: w266 -> [w331]
          tunnel: w264 -> [w328]
          i -> [w329]
          n120 = for {
            N: 4 -> [_]
            tunnel: w331 -> [w375]
            tunnel: w337 -> [w379]
            tunnel: w330 -> [w373]
            tunnel: w336 -> [w352] mode=indexing
            tunnel: [w372] -> w335
            tunnel: [w371] -> w334
            tunnel: [w359] -> w333
            tunnel: w332 -> [w367]
            tunnel: w329 -> [w346]
            tunnel: w328 -> [w340]
            i -> [w358]
            n121 = Multiply(x=w346, y=4) -> (x*y=w343:i32)
            n122 = Increment(x=w358) -> (x+1=w344:i32)
            n123 = Add(x=w343, y=w344) -> (x+y=w342:i32)
            "corner index" <- w342
            n124 = Index Array(array=w352, index=2) -> (element=w350:dbl)
            n125 = flat-sequence {
              tunnel: w379 -> [w419]
              tunnel: [w419] -> w380
              tunnel: w380 -> [w422]
              tunnel: [w422] -> w378
              tunnel: [w421] -> w376
              tunnel: [w420] -> w377
              frame #0 {
              }
              frame #1 {
                n126 = call "air pressure setting.vi"() -> ("air pressure indecator"=w421:i32, "deposit speed 2"=w420:dbl)
              }
            }
            n127 = case shown="8" w342 {
              tunnel: [dbl[] [-2.158, -0.64, 0.0, 0.0] ("distances") dbl[] [-2.196, -0.521, 0.0, 0.0] ("distances") dbl[] [1.449, -0.438, 0.0, 0.0] ("distances") dbl[] [1.217, -0.563, 0.0, 0.0] ("distances") dbl[] [-2.198, -0.263, 0.0, 0.0] ("distances") dbl[] [-2.02, -0.187, 0.0, 0.0] ("distances") dbl[] [1.449, -0.186, 0.0, 0.0] ("distances") dbl[] [1.381, -0.3, 0.0, 0.0] ("distances")] -> w364
              tunnel: [dbl[][] [[3.552, 0.733], [7.0, 0.0], [0.0, -206.0], [-7.0, 0.0]] ("distances") dbl[][] [[3.557, -0.3], [7.0, 0.0], [0.0, -206.0], [-7.0, 0.0]] ("distances") dbl[][] [[-3.736, -0.48], [7.0, 0.0], [0.0, -206.0], [-7.0, 0.0]] ("distances") dbl[][] [[-3.512, 0.563], [7.0, 0.0], [0.0, -206.0], [-7.0, 0.0]] ("distances") dbl[][] [[3.616, 0.287], [7.0, 0.0], [0.0, -206.0], [-7.0, 0.0]] ("distances") dbl[][] [[3.453, -0.694], [7.0, 0.0], [0.0, -206.0], [-7.0, 0.0]] ("distances") dbl[][] [[-3.647, -0.637], [7.0, 0.0], [0.0, -206.0], [-7.0, 0.0]] ("distances") dbl[][] [[-3.66, 0.357], [7.0, 0.0], [0.0, -206.0], [-7.0, 0.0]] ("distances")] -> w363
              frame 1, Default {
              }
              frame 2 {
              }
              frame 3 {
              }
              frame 4 {
                # "Y"
                # "X"
              }
              frame 5 {
              }
              frame 6 {
              }
              frame 7 {
              }
              frame 8 {
              }
            }
            n128 = Add(x=w364, y=w352) -> (x+y=w366:dbl[])
            n129 = Add(x=w367, y=w366) -> (x+y=w365:dbl[])
            n130 = Array Subset(array=w365, index=0, length=2) -> (w368:dbl[])
            "x+y" <- w368
            n131 = call-dynamic "XY Go.vi"("error in (no error)"=w373, "Speed"=80.0, "XY"=w368, "Motion in"=w375) -> ("error out"=w355:errorcluster, "Motion out"=w357:refnum<class "Motion.lvclass">)  [unwired: 6 in]
            n132 = Subtract(x=5.5818 ("y"), y=w340) -> (x-y=w339:dbl)
            n133 = Add(x=w350, y=w339) -> (x+y=w347:dbl)
            n134 = call-dynamic "Z Go.vi"("error in (no error)"=w355, "Speed"=5.0, "Position"=w347, "Motion in"=w357) -> ("error out"=w354:errorcluster, "Motion out"=w356:refnum<class "Motion.lvclass">)  [unwired: 6 in]
            n135 = flat-sequence {
              tunnel: w354 -> [w389]
              tunnel: w356 -> [w388]
              tunnel: [w385] -> w349
              tunnel: [w386] -> w348
              tunnel: w347 -> [w382]
              tunnel: w378 -> [w398]
              tunnel: w377 -> [w397]
              tunnel: w376 -> [w396]
              tunnel: w363 -> [w391]
              tunnel: [w393] -> w362
              tunnel: [w392] -> w361
              tunnel: [w390] -> w360
              tunnel: w349 -> [w394]
              tunnel: w348 -> [w390]
              tunnel: [w401] -> w371
              tunnel: [w402] -> w372
              tunnel: w362 -> [w402]
              tunnel: w361 -> [w401]
              tunnel: w360 -> [w400]
              tunnel: [w399] -> w359
              frame #0 {
                n136 = call "?"("error in (no error)"=w389) -> ("error out"=w387:errorcluster)  [unwired: 9 in, 1 out]
                n137 = Subtract(x=w382, y=3.0) -> (x-y=w381:dbl)
                n138 = call-dynamic "Z Go.vi"("error in (no error)"=w387, "Speed"=5.0, "Position"=w381, "Motion in"=w388) -> ("error out"=w386:errorcluster, "Motion out"=w385:refnum<class "Motion.lvclass">)  [unwired: 6 in]
              }
              frame #1 {
                n139 = call "Muliti_XY_dispense_shih.vi"("Pressure"=w396, "Path count"=1, "Speed"=w397, "distances"=w391, "Ultimus V in"=w398, "Motion in"=w394) -> ("Ultimus V out"=w392:refnum<class "Ultimus V2.lvclass">, "Motion out"=w393:refnum<class "Motion.lvclass">)  [unwired: 4 in]
              }
              frame #2 {
                n140 = call "Time Delay5"("error in (no error)"=w400) -> ("error out"=w399:errorcluster)  [unwired: 10 in]
              }
            }
            "Array" <- w352
          }
        }
        n141 = call "XYZTheta Go.vi"("error in (no error)"=w268, "XYZTheta In"=dbl[] [500.0, 1000.0, 0.0, 0.1], "Motion in"=w285) -> ("error out"=w291:errorcluster, "Motion out"=w289:refnum<class "Motion.lvclass">)  [unwired: 6 in, 1 out]
        n142 = call-dynamic "Disconnect.vi"("Ultimus V in"=w284) -> ()  [unwired: 9 in, 1 out]
        n143 = call "Display Message to User3"("error in (no error)"=w291) -> ()  [unwired: 9 in, 2 out]
      }
      event "Deposit Glue for chip": Value Change {
        # "CF height"
        # "surface z offset"
        # "first needle park position\nneedle gap on Z value : 0.5 mm"
        # "Syringe-camera offset"
        n144 = event-data() -> ()  [unwired: 1 in, 6 out]
        n145 = Add(x=14.2 ("element"), y=w431) -> (x+y=w443:dbl)
        n146 = call-poly <vilib>:"Read Delimited Spreadsheet.vi"("file path (dialog if empty)"=path "D:/INTT/V1/Assembly Data/Tool Offsets/Dispense Tip Offset.txt", "number of rows (all:-1)"=-1) -> ("first row"=w472:dbl[])  [unwired: 8 in, 5 out]
        n147 = Index Array(array=w472, index #1=0 ("index"), index #2=1 ("index")) -> (element #1=w467:dbl, element #2=w466:dbl)
        n148 = Build Array(w467, w466, 0.0 ("element"), 0.0 ("element")) -> (w460:dbl[])
        n149 = Array Subset(array=w434, index (row)=0, length (row)=1 ("length")) -> (w437:dbl[][])  [unwired: 2 in]
        n150 = Reshape Array(w437, 4 ("dimension size")) -> (w436:dbl[])
        n151 = Index Array(array=w436, index=2) -> (element=w432:dbl)
        n152 = Add(x=w432, y=w443) -> (x+y=w442:dbl)
        n153 = Build Array(427.051, 722.276, w442, 0.0 ("element")) -> (w441:dbl[])
        "Needle parking position 2" <- w441
        n154 = call "XYZTheta Go.vi"("XYZTheta In"=w441, "Motion in"=w448) -> ("error out"=w449:errorcluster, "Motion out"=w453:refnum<class "Motion.lvclass">)  [unwired: 7 in, 1 out]
        n155 = call "Display Message to User6"("error in (no error)"=w449) -> ("error out"=w454:errorcluster)  [unwired: 9 in, 1 out]
        n156 = case shown="False" w433 {
          tunnel: w434 -> [w478 w487]
          tunnel: [w475 w487] -> _
          frame False {
            n157 = Array Subset(array=w478, index (row)=1 ("index"), length (row)=1 ("length")) -> (w479:dbl[][])  [unwired: 2 in]
            n158 = Array Subset(array=w478, index (row)=0 ("index"), length (row)=1 ("length")) -> (w482:dbl[][])  [unwired: 2 in]
            n159 = Reshape Array(w482, 4 ("dimension size")) -> (w477:dbl[])
            n160 = Reshape Array(w479, 4 ("dimension size")) -> (w476:dbl[])
            n161 = Build Array(w476, w477) -> (w475:dbl[][])
          }
          frame True {
          }
        }
        n162 = call-dynamic "Z Go.vi"("error in (no error)"=w454, "Speed"=20.0, "Position"=0.0, "Motion in"=w453) -> ("error out"=w452:errorcluster, "Motion out"=w451:refnum<class "Motion.lvclass">)  [unwired: 6 in]
        n163 = call "Display Message to User7"("error in (no error)"=w452) -> ("error out"=w450:errorcluster)  [unwired: 9 in, 1 out]
        n164 = call-dynamic "Connect.vi"("Ultimus V in"=refnum<class "Ultimus V2.lvclass"> refnum ("Ultimus V2.lvclass")) -> ("Ultimus V out"=w457:refnum<class "Ultimus V2.lvclass">)  [unwired: 9 in, 1 out]
        n165 = for {
          N: w459 -> [_]
          tunnel: w457 -> [w498]
          tunnel: w460 -> [w493]
          tunnel: [w496] -> w463
          tunnel: [w495] -> _
          tunnel: w450 -> [w491]
          tunnel: [w494] -> w461
          tunnel: w428 -> [w497] mode=indexing
          tunnel: w451 -> [w492]
          tunnel: w429 -> [w489]
          tunnel: w423 -> [w488] mode=indexing
          i -> [w490]
          n166 = for {
            N: 26 -> [_]
            tunnel: w492 -> [w544]
            tunnel: w498 -> [w548]
            tunnel: w491 -> [w542]
            tunnel: w497 -> [w525] mode=indexing
            tunnel: [w541] -> w496
            tunnel: [w540] -> w495
            tunnel: [w532] -> w494
            tunnel: w493 -> [w536]
            tunnel: w490 -> [w519]
            tunnel: w489 -> [w513]
            tunnel: w488 -> [w511] mode=indexing
            i -> [w531]
            (unwired) dbl[][] [[3.552, 0.733], [7.0, 0.0], [0.0, -206.0], [-7.0, 0.0]] ("distances")
            n167 = Multiply(x=w519, y=0) -> (x*y=w516:i32)
            n168 = Increment(x=w531) -> (x+1=w517:i32)
            n169 = Add(x=w516, y=w517) -> (x+y=w515:i32)
            "corner index 2" <- w515
            n170 = Index Array(array=w525, index=2) -> (element=w523:dbl)
            n171 = case shown="14..26" w515 {
              tunnel: [dbl[] [-0.2, 4.5, 0.0, 0.0] ("distances") dbl[] [0.2, 4.5, 0.0, 0.0] ("distances")] -> w533
              frame 1..13, Default {
              }
              frame 14..26 {
              }
            }
            n172 = Add(x=w533, y=w511) -> (x+y=w535:dbl[])
            n173 = Add(x=w536, y=w535) -> (x+y=w534:dbl[])
            n174 = Array Subset(array=w534, index=0, length=2) -> (w537:dbl[])
            "x+y 2" <- w537
            n175 = call-dynamic "XY Go.vi"("error in (no error)"=w542, "Speed"=80.0, "XY"=w537, "Motion in"=w544) -> ("error out"=w528:errorcluster, "Motion out"=w530:refnum<class "Motion.lvclass">)  [unwired: 6 in]
            n176 = flat-sequence {
              tunnel: [w575] -> w547
              tunnel: [w574] -> w545
              tunnel: [w573] -> w546
              tunnel: w548 -> [w575]
              frame #0 {
                n177 = call "air pressure setting.vi"() -> ("air pressure indecator"=w574:i32, "deposit speed 2"=w573:dbl)
              }
            }
            n178 = Subtract(x=5.5818 ("y"), y=w513) -> (x-y=w512:dbl)
            n179 = Add(x=w523, y=w512) -> (x+y=w520:dbl)
            n180 = call-dynamic "Z Go.vi"("error in (no error)"=w528, "Speed"=5.0, "Position"=w520, "Motion in"=w530) -> ("error out"=w527:errorcluster, "Motion out"=w529:refnum<class "Motion.lvclass">)  [unwired: 6 in]
            n181 = call "check"("error in (no error)"=w527) -> ("error out"=w504:errorcluster)  [unwired: 9 in, 1 out]
            n182 = Subtract(x=w520, y=3.0) -> (x-y=w501:dbl)
            n183 = call-dynamic "Z Go.vi"("error in (no error)"=w504, "Speed"=5.0, "Position"=w501, "Motion in"=w529) -> ("error out"=w521:errorcluster, "Motion out"=w522:refnum<class "Motion.lvclass">)  [unwired: 6 in]
            n184 = case shown="1..13, Default" {
              selector: _ -> [_ _]
              frame 1..13, Default {
              }
              frame 14..26 {
              }
            }
            n185 = call "Muliti_XY_dispense_shih.vi"("Pressure"=w545, "Path count"=1, "Speed"=w546, "distances"=dbl[][] [[3.552, 0.733], [7.0, 0.0], [0.0, -206.0], [-7.0, 0.0]], "Ultimus V in"=w547, "Motion in"=w522) -> ("Ultimus V out"=w540:refnum<class "Ultimus V2.lvclass">, "Motion out"=w541:refnum<class "Motion.lvclass">)  [unwired: 4 in]
            n186 = call "Time Delay"("error in (no error)"=w521) -> ("error out"=w532:errorcluster)  [unwired: 10 in]
            n187 = flat-sequence {
              tunnel: _ -> [w557]
              tunnel: _ -> [w556]
              tunnel: [w553] -> w510
              tunnel: [w554] -> w509
              tunnel: _ -> [w550]
              tunnel: _ -> [w566]
              tunnel: _ -> [w565]
              tunnel: _ -> [w564]
              tunnel: _ -> [w559]
              tunnel: [w561] -> w508
              tunnel: [w560] -> w507
              tunnel: [w558] -> w506
              tunnel: w510 -> [w562]
              tunnel: w509 -> [w558]
              tunnel: [w569] -> _
              tunnel: [w570] -> _
              tunnel: w508 -> [w570]
              tunnel: w507 -> [w569]
              tunnel: w506 -> [w568]
              tunnel: [w567] -> _
              frame #0 {
                n188 = call "3"("error in (no error)"=w557) -> ("error out"=w555:errorcluster)  [unwired: 9 in, 1 out]
                n189 = Subtract(x=w550, y=3.0) -> (x-y=w549:dbl)
                n190 = call-dynamic "Z Go.vi"("error in (no error)"=w555, "Speed"=5.0, "Position"=w549, "Motion in"=w556) -> ("error out"=w554:errorcluster, "Motion out"=w553:refnum<class "Motion.lvclass">)  [unwired: 6 in]
              }
              frame #1 {
                n191 = call "Muliti_XY_dispense_shih.vi"("Pressure"=w564, "Path count"=1, "Speed"=w565, "distances"=w559, "Ultimus V in"=w566, "Motion in"=w562) -> ("Ultimus V out"=w560:refnum<class "Ultimus V2.lvclass">, "Motion out"=w561:refnum<class "Motion.lvclass">)  [unwired: 4 in]
              }
              frame #2 {
                n192 = call "Time Delay2"("error in (no error)"=w568) -> ("error out"=w567:errorcluster)  [unwired: 10 in]
              }
            }
          }
        }
        n193 = call "XYZTheta Go.vi"("error in (no error)"=w461, "XYZTheta In"=dbl[] [500.0, 1000.0, 0.0, 0.1], "Motion in"=w463) -> ("error out"=w465:errorcluster, "Motion out"=w462:refnum<class "Motion.lvclass">)  [unwired: 6 in, 1 out]
        n194 = call "Display Message to User5"("error in (no error)"=w465) -> ()  [unwired: 9 in, 2 out]
      }
      event "Needle Alignment": Value Change {
        (unwired) "Needle Alignment in progress ...." ("String")
        # "CF height"
        # "surface z offset"
        # "first needle park position\nneedle gap on Z value : 0.5 mm"
        # "Syringe-camera offset"
        n195 = event-data() -> ()  [unwired: 1 in, 6 out]
        n196 = Array Subset(array=w581, index (row)=0, length (row)=1 ("length")) -> (w584:dbl[][])  [unwired: 2 in]
        n197 = Reshape Array(w584, 4 ("dimension size")) -> (w583:dbl[])
        n198 = Index Array(array=w583, index=2) -> (element=w580:dbl)
        n199 = call-poly <vilib>:"Read Delimited Spreadsheet.vi"("file path (dialog if empty)"=path "D:/INTT/V1/Assembly Data/Tool Offsets/Dispense Tip Offset.txt", "number of rows (all:-1)"=-1) -> ("first row"=w626:dbl[])  [unwired: 8 in, 5 out]
        n200 = Index Array(array=w626, index #1=0 ("index"), index #2=1 ("index")) -> (element #1=w621:dbl, element #2=w620:dbl)
        n201 = Add(x=14.2 ("element"), y=w589) -> (x+y=w591:dbl)
        n202 = Add(x=w580, y=w591) -> (x+y=w590:dbl)
        n203 = Build Array(424.448, 1040.76, w590, 0.0 ("element")) -> (w588:dbl[])
        n204 = Build Array(w621, w620, 0.0 ("element"), 0.0 ("element")) -> (w598:dbl[])
        n205 = call "XYZTheta Go.vi"("XYZTheta In"=w588, "Motion in"=w613) -> ("error out"=w619:errorcluster, "XYZTheta Out"=w603:dbl[], "Motion out"=w612:refnum<class "Motion.lvclass">)  [unwired: 7 in]
        n206 = call "Display Message to User10"("error in (no error)"=w619) -> ("error out"=w616:errorcluster)  [unwired: 9 in, 1 out]
        n207 = call-dynamic "Z Go.vi"("error in (no error)"=w616, "Speed"=20.0, "Position"=0.0, "Motion in"=w612) -> ("Motion out"=w611:refnum<class "Motion.lvclass">)  [unwired: 6 in, 1 out]
        n208 = Replace Array Subset(array=w603, new element=0.0 ("new element/subarray"), index=2) -> (w600:dbl[])
        n209 = call "Joystick and Camera SHIH VPC- external Connection.vi"("Motion in"=w611, "XYZTheta"=w600, "Measurement Point"="Touch Needle on a surface") -> ("Motion out"=w609:refnum<class "Motion.lvclass">, "Gantry"=w599:dbl[])  [unwired: 4 in, 2 out]
        n210 = Subtract(x=w599, y=w598) -> (x-y=w597:dbl[])
        n211 = call "Joystick and Camera SHIH VPC- external Connection.vi"("Motion in"=w609, "XYZTheta"=w597, "Measurement Point"="Measure the touch spot with camera") -> ("Motion out"=w605:refnum<class "Motion.lvclass">, "Gantry"=w608:dbl[])  [unwired: 4 in, 2 out]
        n212 = Subtract(x=w599, y=w608) -> (x-y=w607:dbl[])
        n213 = call-poly <vilib>:"Write Delimited Spreadsheet.vi"("file path (dialog if empty)"=path "D:/INTT/V1/Assembly Data/Tool Offsets/Dispense Tip Offset.txt", "1D data"=w607, "append to file? (new file:F)"=FALSE) -> ()  [unwired: 11 in, 2 out]
      }
      event "GOTO": Value Change {
        (unwired) "GOING to a position" ("String")
        n214 = event-data() -> ()  [unwired: 1 in, 6 out]
        n215 = call "XYZTheta Go.vi"("XYZTheta In"="Parking position", "Motion in"=w637) -> ("Motion out"=w635:refnum<class "Motion.lvclass">)  [unwired: 7 in, 2 out]
      }
      event "READ Position": Value Change {
        n216 = event-data() -> ()  [unwired: 1 in, 6 out]
        n217 = call-dynamic "Get Current Position.vi"("Motion in"=w651) -> ("XYZTheta Out"=→"Gantry current position":dbl[], "Motion out"=w650:refnum<class "Motion.lvclass">)  [unwired: 8 in, 1 out]
      }
      event Timeout {
        n218 = event-data() -> ()  [unwired: 1 in, 3 out]
        n219 = call-dynamic "Digital Read 1 Channel.vi"("NI-DAQ in"=w661) -> ("NI-DAQ out"=w660:refnum<class "NI-DAQ.lvclass">)  [unwired: 8 in, 2 out]
      }
    }
    "Stave mark" <- w27
    "Sample on HDI" <- w13
    "Measured HDI top left mark" <- w11
    "Measured HDI size" <- w10
    n220 = feedback-in #1(w11) -> ()
    n221 = feedback-in #2(w10) -> ()
    n222 = feedback-in #3(w27) -> ()
    n223 = feedback-in #4(w32) -> ()
    n224 = feedback-in #5(w20) -> ()
    n225 = feedback-in #6(w35) -> ()
    n226 = feedback-in #7(w18) -> ()
    n227 = feedback-in #8(w13) -> ()
    n228 = feedback-in #9(w9) -> ()
    "# of tasks excuted" <- w33
  }
  n229 = call-dynamic "Disconnect.vi"("Controller in"=w4) -> ()  [unwired: 9 in, 1 out]
  n230 = call-dynamic "Disconnect.vi"("I-O in"=w1) -> ()  [unwired: 9 in, 1 out]
